vi "Pagina sinottico.vi"() -> (0 "pagina out":i16=255)   [LabVIEW 2022 SP3]
uses:
  Labview/Globali.vi
  <vilib>/Utility/inputDevices.llb/closeKeyboard.vi
  <vilib>/Utility/inputDevices.llb/keyboardAcquire.vi
panel:
  in  "solo a macchina ferma e ciclo concluso":bool
  out "CARRO IN POSIZIONE RP3000":bool
  out "CARRO IN POSIZIONE AAT":bool
  out "PRESSURIZZAZIONE":sgl(slide) caption="Pressurizz.\n\n[bar]" scale=0.0..1.0 scale format="%.1f"
  out "PRESSIONE ARIA 6 BAR":sgl(slide) caption="Pressione\n\n[bar]" scale=0.0..10.0
  out "PORTATA RICIRCOLO":sgl(slide) caption="Portata\nricircolo\n[l/min]" scale=0.0..25.0
  out "Cicli macchina":u16 caption="TIMEOUT\nMANUTENZIONE"
  in  "Vi/NaSH+F2":bool
  in  "Continua prova":bool
  in  "SOSPENDI PROVA":bool
  out "TEMPERATURA OLIO 10W30":sgl(slide) caption="Temperatura olio 10W30 [°C]" scale=0.0..100.0
  out "TEMPERATURA OLIO W90":sgl(slide) caption="Temperatura olio W90 [°C]" scale=0.0..100.0
  out "Rotaz.SX":bool
  out "Rotaz.DX":bool
  out "VELOCITA' MOTORE":u16(knob) caption="Velocità\n[rpm]" scale=0.0..3000.0
  out "Serial Number":string
  out "Prodotto":string
  in  "ANNULLA PROVA":bool
  out "S_AUTO":bool
  in  "0. 1":bool
  out "AVANZAMENTO COLLAUDO":i8(slide) scale=0.0..8.0
  out "t. 7":i32=17395251 format="%<%H:%M:%S>t"
  out "t. 6":i32=17395251 format="%<%H:%M:%S>t"
  out "t. 5":i32=17395251 format="%<%H:%M:%S>t"
  out "t. 4":i32=17395251 format="%<%H:%M:%S>t"
  out "t. 3":i32=17395251 format="%<%H:%M:%S>t"
  out "t. 2":i32=17395251 format="%<%H:%M:%S>t"
  out "t. 1":i32=17395251 format="%<%H:%M:%S>t"
  in  "t. 0":i32=17395251 format="%<%H:%M:%S>t"
  in  "Si/No 9":cluster{"Si":bool, "No":bool}
  in  "Si/No 8":cluster{"Si":bool, "No":bool}
  in  "Si/No 7":cluster{"Si":bool, "No":bool}
  in  "Si/No 6":cluster{"Si":bool, "No":bool}
  in  "Si/No 5":cluster{"Si":bool, "No":bool}
  in  "Si/No 4":cluster{"Si":bool, "No":bool}
  in  "Si/No 3":cluster{"Si":bool, "No":bool}
  in  "Si/No 2":cluster{"Si":bool, "No":bool}
  in  "Si/No 1":cluster{"Si":bool, "No":bool}
  out "t. tot.":i32 format="%<%H:%M:%S>t"
  out "t. Step":i32 format="%<%H:%M:%S>t"
  out "Indicazioni":string="Operatore:\t\t\t\t\t\t\t\t\t\t\t\t\t\t\t\t\t\t\t\t\t\t\t\t\t\t\t\t\t\t\t\tPart number:\t\t\t\t\t\t\t\t\t\t\t\t\t\t\t\t\t\t\t\t\t\t\t\t\t\t\t\t\t\t\t\tMatricola:\t\t\t\t\t\t\t\t\t\t\t\t\t\t\t\t0\t\t\t\t\t\t\t\t\t\t\t\t\t\t\t\tStatus \t\t\t\t\t\t\t\t\t\t\t\t\t\t\t\tC:\\Documents and Settings\\IVECO\\Reports\\\\"
  out "Prova":bool=TRUE
  in  "Login":bool
  in  "stop":bool
  in  "Comandi manuali":bool
  out "Picture":picture
  out "Versione SW":dbl=2.0 format="%.2f"
  out "Linea":string="BANCO PROVA TENUTA"
  out "Tipo pagina":string="PROVA"
  out "PRESSIONE RICIRCOLO":sgl(slide) caption="Pressione\nricircolo\n[bar]" scale=0.0..2.5 scale format="%.1f"
  out "TEMPERATURA CUSCIN.":sgl(slide) caption="Temperatura\ncuscinetto\n[°C]" scale=0.0..120.0
  out "TEMPERATURA OLIO COPPA":sgl(slide) caption="Temperatura\nolio coppa\n[°C]" scale=0.0..120.0
  out "COPPIA ASSE":sgl(knob) caption="Coppia\n[Nm]" scale=0.0..100.0
  out "Trazione inserita":bool
  out "PROT35":bool
  out "W90":bool
  out "10W30":bool
  in  "2. 5":bool
  in  "1. 3":bool
  in  "2. 0":bool
  in  "2. 3":bool
  in  "1. 4":bool
  in  "1. 5":bool
  in  "1. 6":bool
  in  "1. 7":bool
  in  "2. 1":bool
  in  "2. 2":bool
  in  "2. 4":bool
  out "TEMPERATURA AMBIENTE":sgl(slide) caption="Temperatura\nambiente\n[°C]" scale=0.0..50.0
  in  "1. 1":bool
  in  "1. 2":bool
  in  "0. 7":bool
  in  "1. 0":bool
  in  "0. 5":bool
  in  "0. 6":bool
  in  "0. 2":bool
  in  "0. 3":bool
  in  "0. 4":bool
  out "Testo allarmi":string caption="ALLARMI"
  out "Testo fase collaudo":string caption="FASE COLLAUDO"
  out "Testo segnalazioni":string caption="SEGNALAZIONI"
  out "Testo messaggi":string caption="MESSAGGI"
  out "forza chiusura":bool
  out "PLC->PC":string[](array[string])
  out "COD.PRODOTTO":string
  out "CODICE":string
  out "MATRICOLA OPERATORE":string
  in  "Pagina misure":bool
  in  "stop 2":bool
  in  "Pagina diagnostica":bool
  in  "Pagina scarti":bool
  out "Nome File Dati":string="C:\\Documents and Settings\\IVECO\\Reports\\\\"
  in  "Pagina parametri":bool
  out "operazioni":string[][](table)
  # "MODO FUNZIONAMENTO"
  # "INSERIMENTO TRAZIONE"
  # "SELETTORE SCARICO"
  # "OPERAZIONE"
  # "RICIRCOLO OLIO"
  # "CARICO/SCARICO PRESSURIZZAZIONE"
  # "CARICO/SCARICO ARIA"
  # "MOTORE"
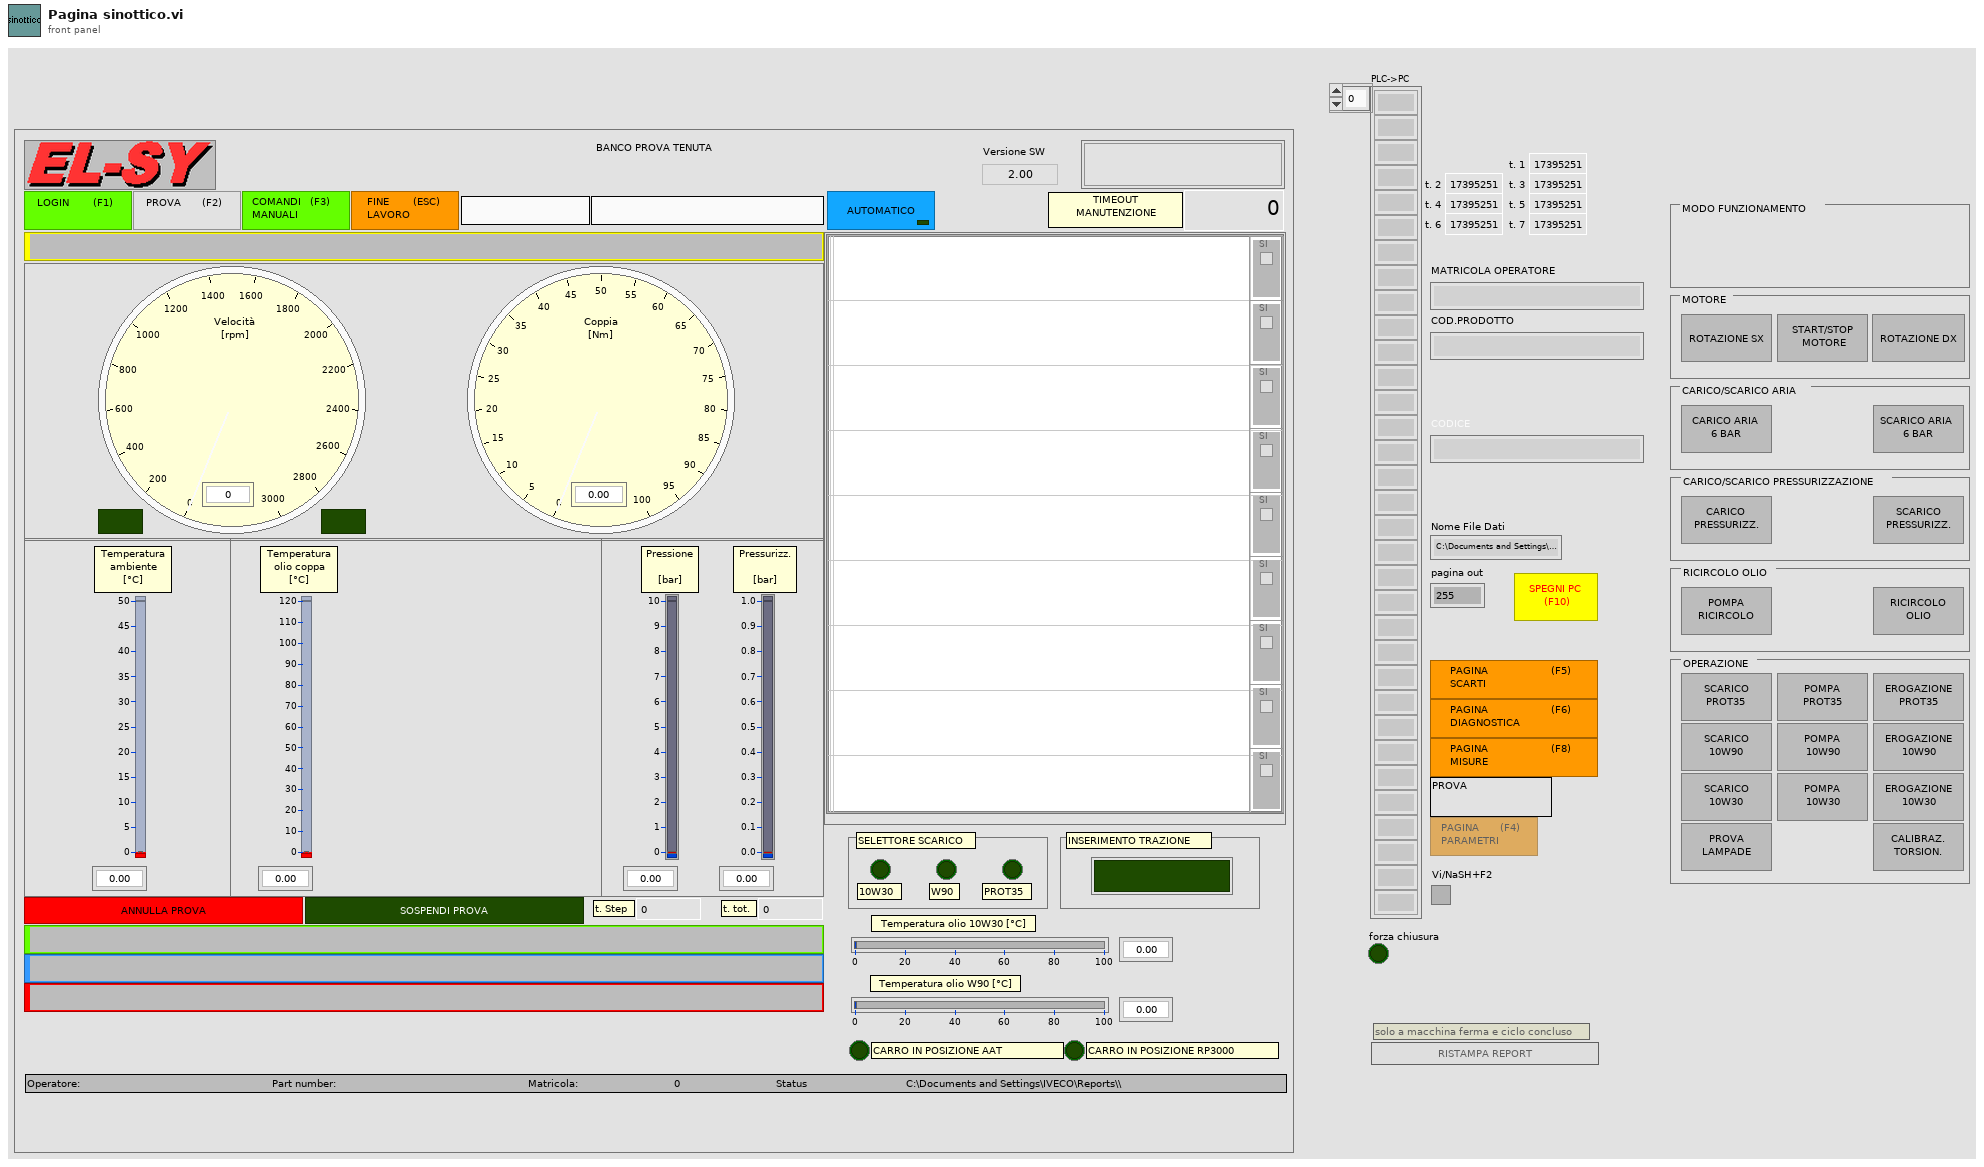
[diagram p1: front panel]
types:
  T1 = enum16{"0", "1", "2", "3", "4", "5", "6", "7", "8", "9", "A", "B", "C", "D", "E", "F", "G", "H", "I", "J", "K", "L", "M", "N", "O", "P", "Q", "R", "S", "T", "U", "V", "W", "X", "Y", "Z", "F1", "F2", "F3", "F4", "F5", "F6", "F7", "F8", "F9", "F10", "F11", "F12", "F13", "F14", "F15", "ADD", "BACK", "BACKSLASH", "CAPITAL", "COMMA", "DECIMAL", "DELETE", "DIVIDE", "DOWN", "END", "EQUALS", "ESCAPE", "GRAVE (`)", "HOME", "INSERT", "LBRACKET", "LCONTROL", "LEFT", "L ALT", "LSHIFT", "LWIN", "MINUS", "MULTIPLY", "NEXT", "NUMLOCK", "NUMPAD_0", "NUMPAD_1", "NUMPAD_2", "NUMPAD_3", "NUMPAD_4", "NUMPAD_5", "NUMPAD_6", "NUMPAD_7", "NUMPAD_8", "NUMPAD_9", "PAUSE", "PERIOD", "PRIOR (PG UP)", "RBRACKET", "RCONTROL", "RETURN", "RIGHT", "R ALT", "RSHIFT", "RWIN", "SCROLL", "SEMICOLON", "SLASH", "SPACE", "SUBTRACT", "TAB", "UP", "ENTER (num pad)", "' (quote)"}[]
  T2 = cluster{"Disable?":i16, "Si":bool, "No":bool, "Dis. No?":i16}
  T3 = enum16{"0", "1", "2", "3", "4", "5", "6", "7", "8", "9", "A", "B", "C", "D", "E", "F", "G", "H", "I", "J", "K", "L", "M", "N", "O", "P", "Q", "R", "S", "T", "U", "V", "W", "X", "Y", "Z", "F1", "F2", "F3", "F4", "F5", "F6", "F7", "F8", "F9", "F10", "F11", "F12", "F13", "F14", "F15", "ADD", "BACK", "BACKSLASH", "CAPITAL", "COMMA", "DECIMAL", "DELETE", "DIVIDE", "DOWN", "END", "EQUALS", "ESCAPE", "GRAVE (`)", "HOME", "INSERT", "LBRACKET", "LCONTROL", "LEFT", "L ALT", "LSHIFT", "LWIN", "MINUS", "MULTIPLY", "NEXT", "NUMLOCK", "NUMPAD_0", "NUMPAD_1", "NUMPAD_2", "NUMPAD_3", "NUMPAD_4", "NUMPAD_5", "NUMPAD_6", "NUMPAD_7", "NUMPAD_8", "NUMPAD_9", "PAUSE", "PERIOD", "PRIOR (PG UP)", "RBRACKET", "RCONTROL", "RETURN", "RIGHT", "R ALT", "RSHIFT", "RWIN", "SCROLL", "SEMICOLON", "SLASH", "SPACE", "SUBTRACT", "TAB", "UP", "ENTER (num pad)", "' (quote)"}
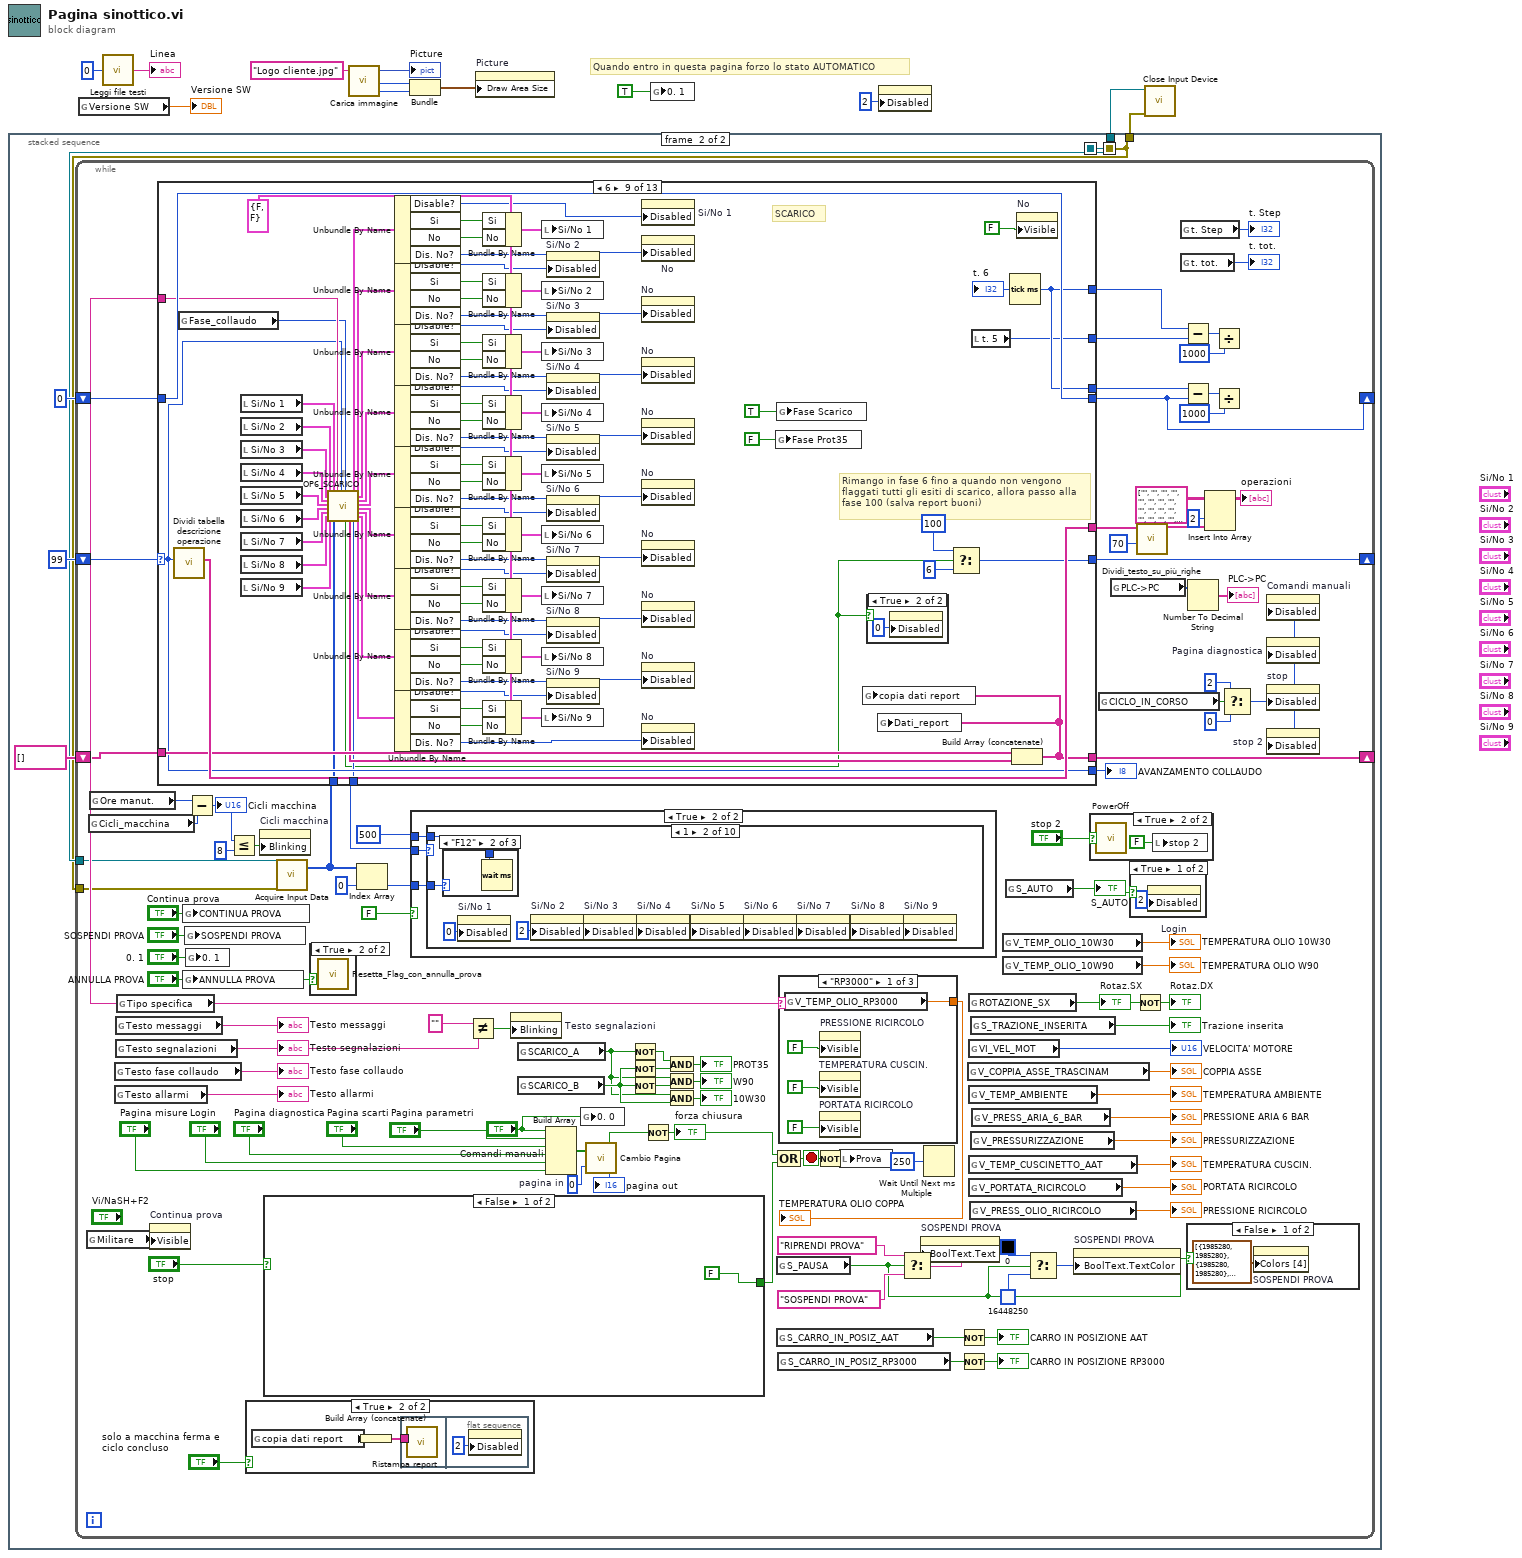
[diagram p0: block diagram]
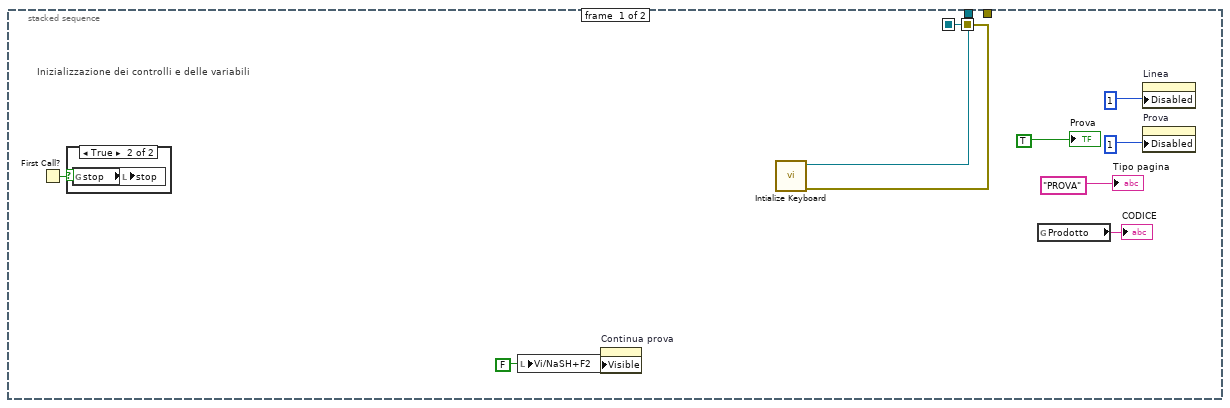
[diagram p2: hidden frame]
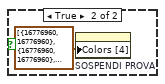
[diagram p5: hidden frame]
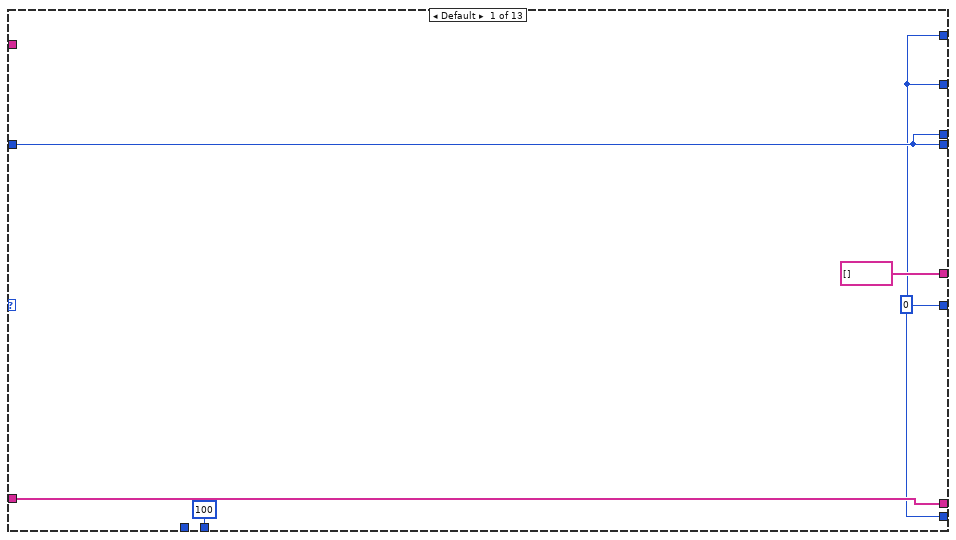
[diagram p6: hidden frame]
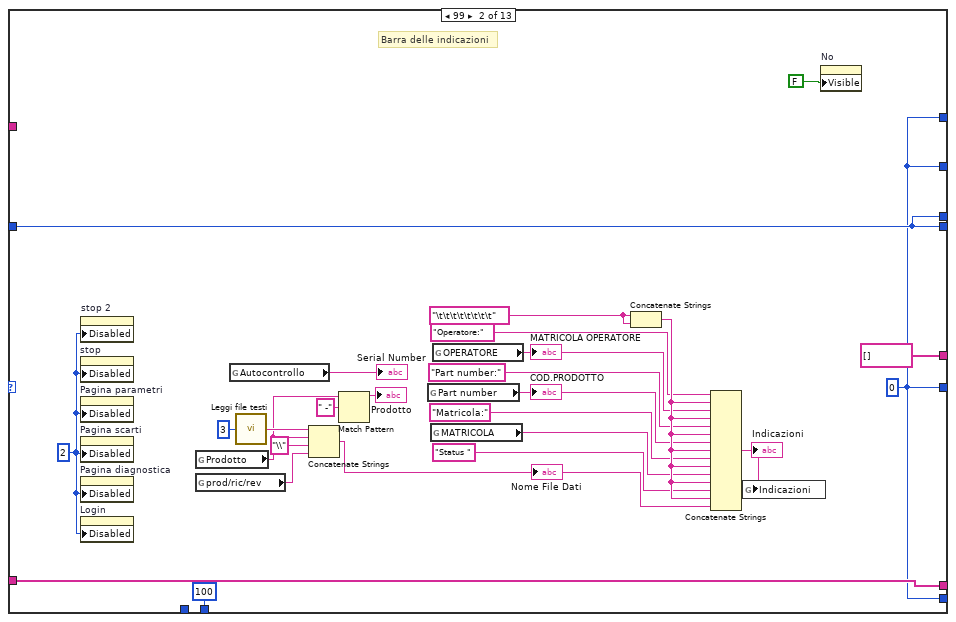
[diagram p7: hidden frame]
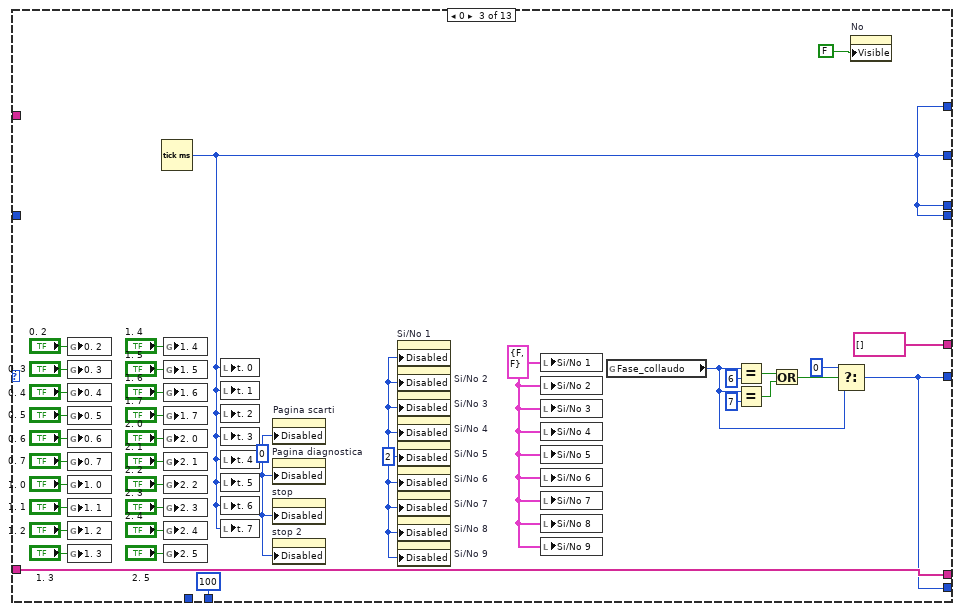
[diagram p8: hidden frame]
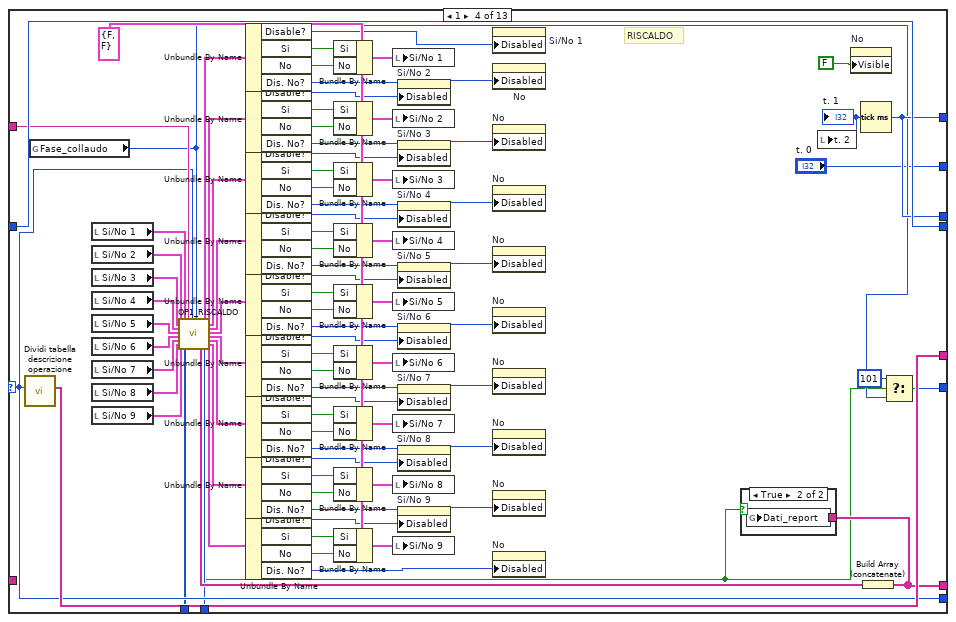
[diagram p9: hidden frame]
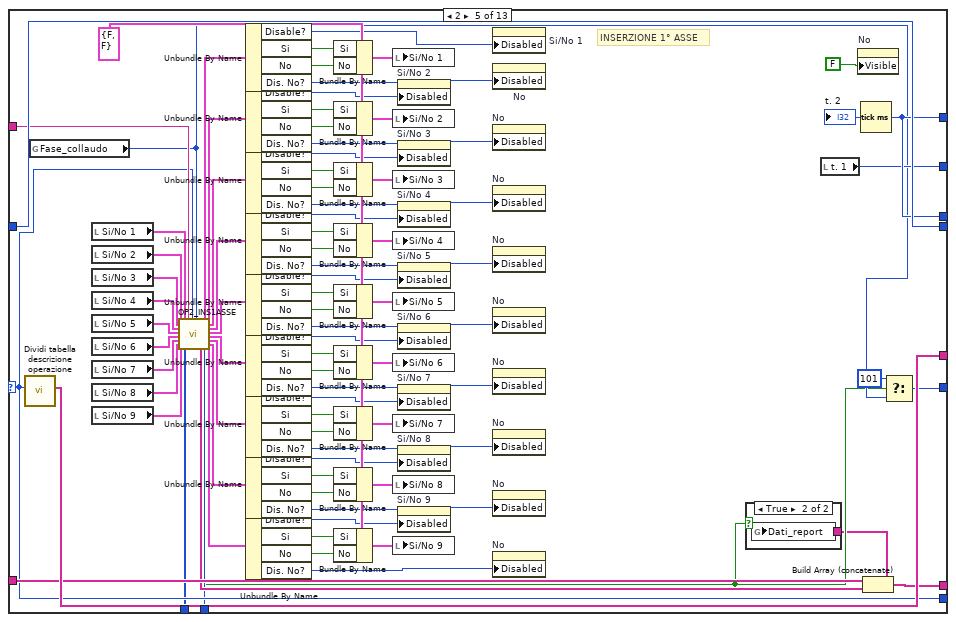
[diagram p11: hidden frame]
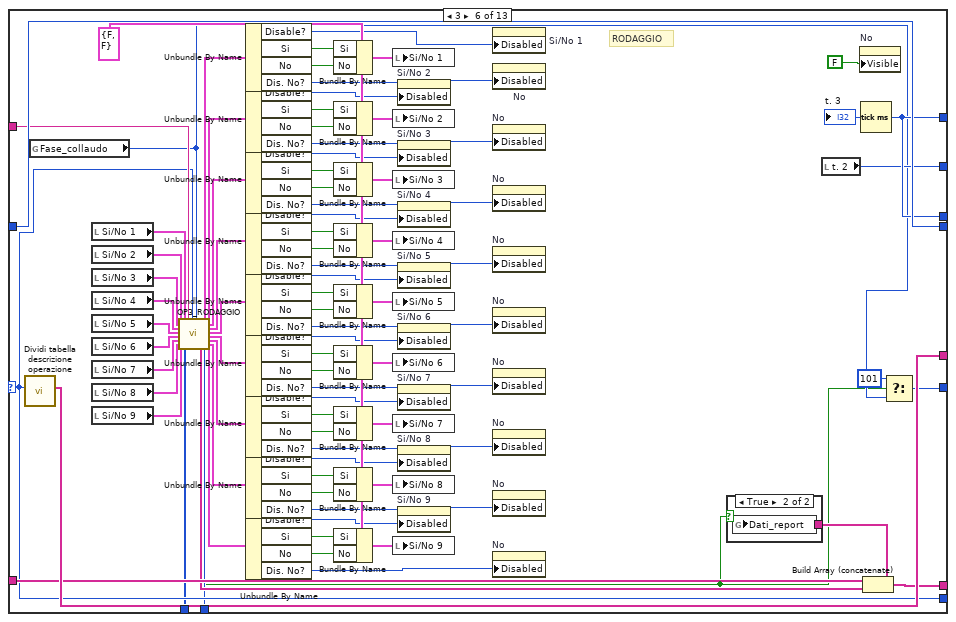
[diagram p13: hidden frame]
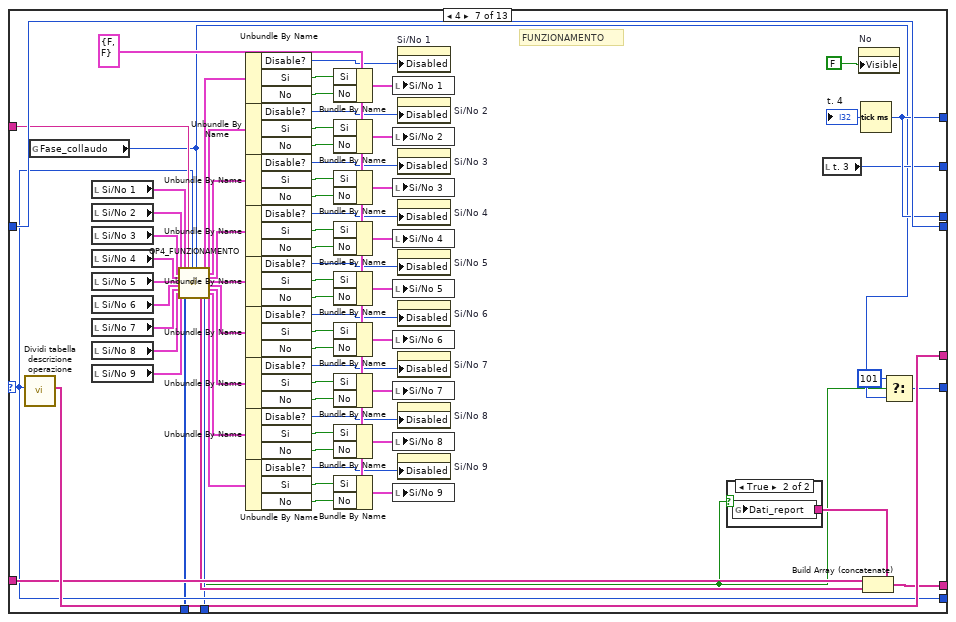
[diagram p15: hidden frame]
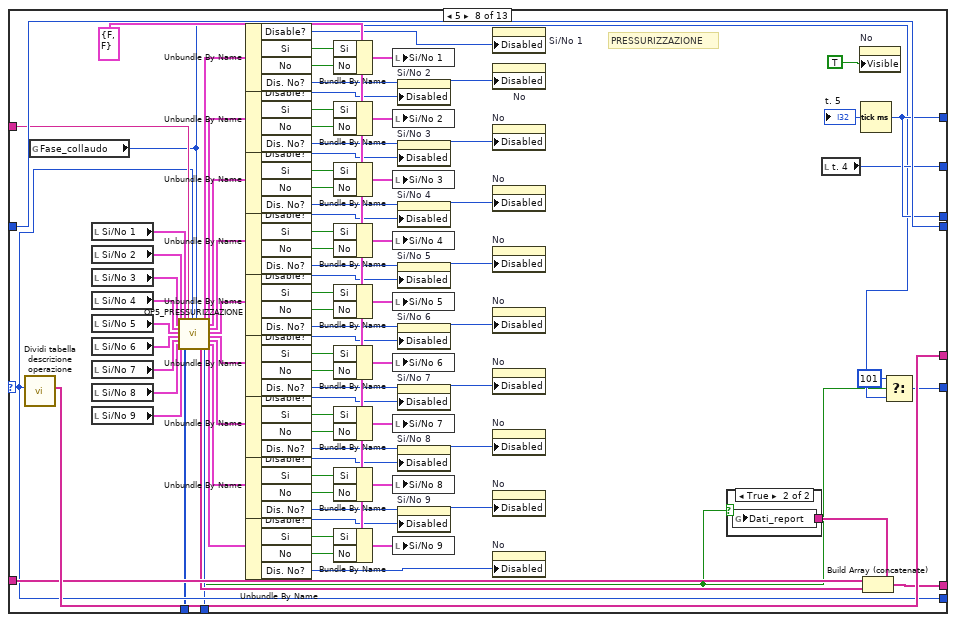
[diagram p17: hidden frame]
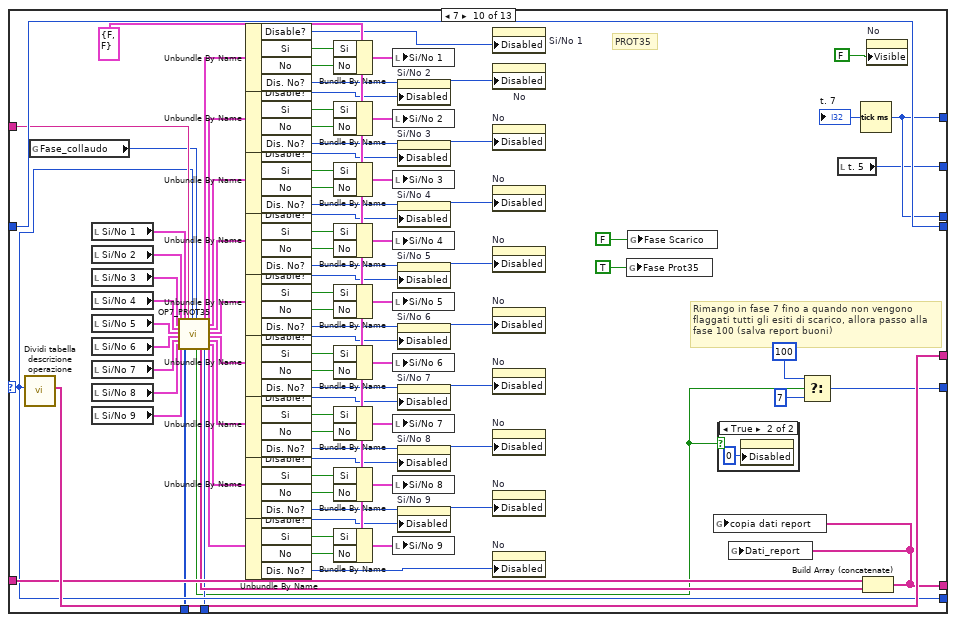
[diagram p20: hidden frame]
diagram:
  # "Quando entro in questa pagina forzo lo stato AUTOMATICO"
  n1 = stacked-sequence {
    seq-local: [w16 _] -> [_ w24]
    seq-local: [w15 _] -> [_ w23]
    tunnel: [_ w23] -> w12
    tunnel: [_ w24] -> w11
    frame #0 {
      w13 = FALSE ("Vi/NaSH+F2")
      # "Inizializzazione dei controlli e delle variabili"
      n2 = First Call?() -> (First Call?: T/F=w21:bool)
      n3 = case shown="True" w21 {
        frame False {
        }
        frame True {
          n4 = global read "Globali.vi" "stop"() -> (w22:bool)
          n5 = local write "stop"(w22) -> ()
        }
      }
      n6 = local write "Vi/NaSH+F2"(w13) -> ()
      n7 = property on="Continua prova" class="Bool (strict)"("Visible"=w13) -> ()  [unwired: 2 in, 2 out]
      n8 = call <vilib>:"Intialize Keyboard.vi"() -> ("error out"=w15:errorcluster, "device ID"=w16:refnum<k1>)  [unwired: 10 in]
      n9 = global read "Globali.vi" "Prodotto"() -> (→"CODICE":string)
      n10 = property on="Linea" class="Str"("Disabled"=u8 1) -> ()  [unwired: 2 in, 2 out]
      n11 = property on="Prova" class="Bool"("Disabled"=u8 1) -> ()  [unwired: 2 in, 2 out]
      "Prova" <- TRUE ("Pagina sinottico")
      "Tipo pagina" <- "PROVA" ("Tipo pagina")
    }
    frame #1 {
      n12 = while {
        shift-right: [w103] -> _
        shift-left: 99 ("Fase_collaudo") -> [w132]
        shift-right: [w101] -> _
        shift-left: u32 0 ("millisecond timer value") -> [w102]
        shift-right: [w96] -> _
        shift-left: string[] [] -> [w95]
        tunnel: w24 -> [w90]
        tunnel: w23 -> [w89]
        stop <- w105 stop-if-true
        w129 = u8 0  # pagina in
        n13 = global read "Globali.vi" "Militare"() -> (w45:bool)
        n14 = global read "Globali.vi" "Cicli_macchina"() -> (w39:u16)
        n15 = global read "Globali.vi" "Ore manut."() -> (w40:i16)
        n16 = global read "Globali.vi" "Testo fase collaudo"() -> (→"Testo fase collaudo":string)
        n17 = global read "Globali.vi" "Testo allarmi"() -> (→"Testo allarmi":string)
        n18 = global read "Globali.vi" "Testo messaggi"() -> (→"Testo messaggi":string)
        n19 = global read "Globali.vi" "Testo segnalazioni"() -> (w30:string)
        "Testo segnalazioni" <- w30
        n20 = global read "Globali.vi" "Tipo specifica"() -> (w97:string)
        n21 = property on="Continua prova" class="Bool (strict)"("Visible"=w45) -> ()  [unwired: 2 in, 2 out]
        n22 = global write "Globali.vi" "CONTINUA PROVA"("Continua prova") -> ()
        n23 = global write "Globali.vi" "ANNULLA PROVA"("ANNULLA PROVA") -> ()
        n24 = global write "Globali.vi" "SOSPENDI PROVA"("SOSPENDI PROVA") -> ()
        n25 = global write "Globali.vi" "0. 1"("0. 1") -> ()
        n26 = Subtract(x=w40, y=w39) -> (x-y=w38:u16)
        "Cicli macchina" <- w38
        n27 = Less Or Equal?(x=w38, y=u16 8) -> (x <= y?=w36:bool)
        n28 = case shown="True" "solo a macchina ferma e ciclo concluso" {
          frame False {
          }
          frame True {
            n29 = global read "Globali.vi" "copia dati report"() -> (w134:string[])
            n30 = Build Array (concatenate)(w134) -> (w133:string[])
            n31 = flat-sequence {
              tunnel: w133 -> [w135]
              frame #0 {
                n32 = call "Ristampa report.vi"("Dato"=w135) -> ()  [unwired: 7 in, 2 out]
              }
              frame #1 {
                n33 = property on="solo a macchina ferma e ciclo concluso" class="Bool"("Disabled"=u8 2) -> ()  [unwired: 2 in, 2 out]
              }
            }
          }
        }
        n34 = property on="Cicli macchina" class="DigNum (strict)"("Blinking"=w36) -> ()  [unwired: 2 in, 2 out]
        n35 = case shown="False" "stop" {
          tunnel: [FALSE ("x = y?") w893] -> w122
          frame False {
          }
          frame True {
            # "Quando esco dal programma forzo lo stato MANUALE"
            n36 = Two Button Dialog(message="USCIRE DALL'APPLICAZIONE?" ("T button name (\"OK\")"), 1:"NO" ("F button name (\"Cancel\")"), 2:"SI" ("T button name (\"OK\")")) -> (T button?=w896:bool)
            n37 = Select(t=TRUE, s=w896, f=FALSE) -> (s? t:f=w894:bool)
            n38 = case shown="True" w894 {
              tunnel: [FALSE ("S_MAN") w902] -> w893
              frame False {
              }
              frame True {
                n39 = while {
                  tunnel: [w903] -> w902
                  stop <- w903 stop-if-true
                  n40 = global read "Globali.vi" "S_MAN"() -> (w903:bool)
                  n41 = Wait Until Next ms Multiple(millisecond multiple=u32 50) -> ()  [unwired: 1 out]
                }
              }
            }
            n42 = global write "Globali.vi" "0. 0"(w894) -> ()
            n43 = local write "stop"(w894) -> ()
            n44 = Quit LabVIEW(quit? (T)=w893) -> ()
            n45 = global write "Globali.vi" "stop"(w893) -> ()
          }
        }
        n46 = call-poly <vilib>:"Acquire Input Data.vi"("device ID"=w90, "error in (no error)"=w89) -> ("keys pressed"=w87:T1)  [unwired: 15 in, 2 out]
        n47 = case shown="6" w132 {
          selector: w132 -> [_ _ _ w215 w294 w375 w456 w528 w610 w695 _ _ _]
          tunnel: [w140 w153 w172 w211 w289 w370 w451 w523 w604 w687 w774 w797 w815] -> w103
          tunnel: [w140 w153 w179 w216 w296 w377 w458 w530 w612 w697 w783 w806 w815] -> w73
          tunnel: [w140 w153 w179 "t. 0" w295 w376 w457 w529 w611 w696 w777 w800 w815] -> w61
          tunnel: [string[] [] string[] [] string[] [] w246 w327 w408 w480 w561 w645 w729 string[] [] string[] [] string[] [] ("operazioni")] -> w64
          tunnel: [w142 w167 w179 w247 w328 w409 w481 w562 w646 w730 w784 w807 w816] -> w101
          tunnel: w102 -> [w142 w167 _ w247 w328 w409 w481 w562 w646 w730 w784 w807 w816]
          tunnel: [w142 w167 w179 w216 w296 w377 w458 w530 w612 w697 w783 w806 w816] -> w65
          tunnel: w97 -> [_ _ _ w236 w317 w398 w470 w551 w635 w719 w769 w792 _]
          tunnel: [w141 w166 w184 w207 w286 w368 w449 w521 w605 w691 w772 w795 w818] -> w96
          tunnel: w95 -> [w141 w166 w184 _ w298 w379 w460 w532 w616 w699 _ _ w818]
          tunnel: [w140 w153 w172 w215 w294 w375 w456 w528 w610 w695 8 ("Fase_collaudo") 8 ("Fase_collaudo") w815] -> w60
          tunnel: [100 ("i out") 100 ("i out") 100 ("i out") w214 w293 w373 w455 w527 w609 w694 100 ("i out") 100 ("i out") 100 ("i out")] -> w88
          tunnel: w87 -> [_ _ _ w213 w292 w374 w454 w526 w608 w693 _ _ _]
          frame Default {
            w140 = 0
          }
          frame 99 {
            w163 = "\t\t\t\t\t\t\t\t" ("String")
            w169 = u8 2 ("Disabled")
            w153 = 0
            # "Barra delle indicazioni"
            n48 = property on="stop 2" class="Bool (strict)"("Disabled"=w169) -> ()  [unwired: 2 in, 2 out]
            n49 = property on="stop" class="Bool (strict)"("Disabled"=w169) -> ()  [unwired: 2 in, 2 out]
            n50 = property on="Pagina parametri" class="Bool"("Disabled"=w169) -> ()  [unwired: 2 in, 2 out]
            n51 = property on="Pagina scarti" class="Bool"("Disabled"=w169) -> ()  [unwired: 2 in, 2 out]
            n52 = property on="Pagina diagnostica" class="Bool"("Disabled"=w169) -> ()  [unwired: 2 in, 2 out]
            n53 = property on="Login" class="Bool"("Disabled"=w169) -> ()  [unwired: 2 in, 2 out]
            n54 = global read "Globali.vi" "Prodotto"() -> (w150:string)
            n55 = global read "Globali.vi" "prod/ric/rev"() -> (w146:string)
            n56 = global read "Globali.vi" "Autocontrollo"() -> (→"Serial Number":string)
            n57 = call "Leggi file testi.vi"("Numero riga"=3) -> ("Testo"=w165:string)  [unwired: 3 in, 1 out]
            n58 = Concatenate Strings(w165, w150, "\\" ("string"), w146) -> (w144:string)
            "Nome File Dati" <- w144
            n59 = Match Pattern(string=w150, regular expression=" -") -> (before substring=→"Prodotto":string)  [unwired: 1 in, 3 out]
            n60 = global read "Globali.vi" "Part number"() -> (w161:string)
            "COD.PRODOTTO" <- w161
            n61 = global read "Globali.vi" "MATRICOLA"() -> (w160:string)
            n62 = global read "Globali.vi" "OPERATORE"() -> (w159:string)
            "MATRICOLA OPERATORE" <- w159
            n63 = Concatenate Strings(w163, w163) -> (w162:string)
            n64 = Concatenate Strings("Operatore:" ("string"), w162, w159, w162, "Part number:" ("string"), w162, w161, w162, "Matricola:" ("string"), w162, w160, w162, "Status " ("string"), w162, w144) -> (w154:string)
            "Indicazioni" <- w154
            n65 = global write "Globali.vi" "Indicazioni"(w154) -> ()
            n66 = property on="No" class="Bool (strict)"("Visible"=FALSE) -> ()  [unwired: 2 in, 2 out]
          }
          frame 0 {
            w180 = cluster{"Si":bool, "No":bool} {"Si"=FALSE, "No"=FALSE} ("Si/No 1")
            w182 = u8 0 ("Disabled")
            w183 = 2
            n67 = global write "Globali.vi" "0. 2"("0. 2") -> ()
            n68 = global write "Globali.vi" "0. 3"("0. 3") -> ()
            n69 = global write "Globali.vi" "0. 4"("0. 4") -> ()
            n70 = global write "Globali.vi" "0. 5"("0. 5") -> ()
            n71 = global write "Globali.vi" "0. 6"("0. 6") -> ()
            n72 = global write "Globali.vi" "0. 7"("0. 7") -> ()
            n73 = global write "Globali.vi" "1. 0"("1. 0") -> ()
            n74 = global write "Globali.vi" "1. 1"("1. 1") -> ()
            n75 = global write "Globali.vi" "1. 2"("1. 2") -> ()
            n76 = global write "Globali.vi" "1. 3"("1. 3") -> ()
            n77 = Tick Count (ms)() -> (millisecond timer value=w179:u32)
            n78 = global write "Globali.vi" "1. 4"("1. 4") -> ()
            n79 = global write "Globali.vi" "1. 5"("1. 5") -> ()
            n80 = global write "Globali.vi" "1. 6"("1. 6") -> ()
            n81 = global write "Globali.vi" "1. 7"("1. 7") -> ()
            n82 = global write "Globali.vi" "2. 0"("2. 0") -> ()
            n83 = global write "Globali.vi" "2. 1"("2. 1") -> ()
            n84 = global write "Globali.vi" "2. 2"("2. 2") -> ()
            n85 = global write "Globali.vi" "2. 3"("2. 3") -> ()
            n86 = global write "Globali.vi" "2. 4"("2. 4") -> ()
            n87 = global write "Globali.vi" "2. 5"("2. 5") -> ()
            n88 = local write "t. 0"(w179) -> ()
            n89 = local write "t. 1"(w179) -> ()
            n90 = local write "t. 2"(w179) -> ()
            n91 = local write "t. 3"(w179) -> ()
            n92 = local write "t. 4"(w179) -> ()
            n93 = local write "t. 5"(w179) -> ()
            n94 = local write "t. 6"(w179) -> ()
            n95 = local write "t. 7"(w179) -> ()
            n96 = property on="Pagina scarti" class="Bool"("Disabled"=w182) -> ()  [unwired: 2 in, 2 out]
            n97 = property on="Pagina diagnostica" class="Bool"("Disabled"=w182) -> ()  [unwired: 2 in, 2 out]
            n98 = property on="stop" class="Bool (strict)"("Disabled"=w182) -> ()  [unwired: 2 in, 2 out]
            n99 = property on="stop 2" class="Bool (strict)"("Disabled"=w182) -> ()  [unwired: 2 in, 2 out]
            n100 = property on="Si/No 1" class="Clust (strict)"("Disabled"=w183) -> ()  [unwired: 2 in, 2 out]
            n101 = property on="Si/No 2" class="Clust (strict)"("Disabled"=w183) -> ()  [unwired: 2 in, 2 out]
            n102 = property on="Si/No 3" class="Clust (strict)"("Disabled"=w183) -> ()  [unwired: 2 in, 2 out]
            n103 = property on="Si/No 4" class="Clust (strict)"("Disabled"=w183) -> ()  [unwired: 2 in, 2 out]
            n104 = property on="Si/No 5" class="Clust (strict)"("Disabled"=w183) -> ()  [unwired: 2 in, 2 out]
            n105 = property on="Si/No 6" class="Clust (strict)"("Disabled"=w183) -> ()  [unwired: 2 in, 2 out]
            n106 = property on="Si/No 7" class="Clust (strict)"("Disabled"=w183) -> ()  [unwired: 2 in, 2 out]
            n107 = property on="Si/No 8" class="Clust (strict)"("Disabled"=w183) -> ()  [unwired: 2 in, 2 out]
            n108 = property on="Si/No 9" class="Clust (strict)"("Disabled"=w183) -> ()  [unwired: 2 in, 2 out]
            n109 = local write "Si/No 1"(w180) -> ()
            n110 = local write "Si/No 2"(w180) -> ()
            n111 = local write "Si/No 3"(w180) -> ()
            n112 = local write "Si/No 4"(w180) -> ()
            n113 = local write "Si/No 5"(w180) -> ()
            n114 = local write "Si/No 6"(w180) -> ()
            n115 = local write "Si/No 7"(w180) -> ()
            n116 = local write "Si/No 8"(w180) -> ()
            n117 = local write "Si/No 9"(w180) -> ()
            n118 = global read "Globali.vi" "Fase_collaudo"() -> (w170:u16)
            n119 = Equal?(x=w170, y=u16 6) -> (x = y?=w175:bool)
            n120 = Equal?(x=w170, y=u16 7) -> (x = y?=w174:bool)
            n121 = Or(x=w175, y=w174) -> (x .or. y?=w173:bool)
            n122 = Select(t=u16 0 ("y"), s=w173, f=w170) -> (s? t:f=w172:u16)
            n123 = property on="No" class="Bool (strict)"("Visible"=FALSE) -> ()  [unwired: 2 in, 2 out]
          }
          frame 1 {
            w278 = cluster{"Si":bool, "No":bool} {"Si"=FALSE, "No"=FALSE} ("Si/No 1")
            # "RISCALDO"
            n124 = call "Dividi tabella descrizione operazione.vi"("Numero operazione"=w215) -> ("operazioni"=w246:string[])  [unwired: 10 in]
            n125 = global read "Globali.vi" "Fase_collaudo"() -> (w212:u16)
            n126 = local read "Si/No 1"() -> (w245:cluster{"Si":bool, "No":bool})
            n127 = local read "Si/No 2"() -> (w244:cluster{"Si":bool, "No":bool})
            n128 = local read "Si/No 3"() -> (w243:cluster{"Si":bool, "No":bool})
            n129 = local read "Si/No 4"() -> (w242:cluster{"Si":bool, "No":bool})
            n130 = local read "Si/No 5"() -> (w241:cluster{"Si":bool, "No":bool})
            n131 = local read "Si/No 6"() -> (w237:cluster{"Si":bool, "No":bool})
            n132 = local read "Si/No 7"() -> (w238:cluster{"Si":bool, "No":bool})
            n133 = local read "Si/No 8"() -> (w239:cluster{"Si":bool, "No":bool})
            n134 = local read "Si/No 9"() -> (w240:cluster{"Si":bool, "No":bool})
            n135 = call "OP1_RISCALDO.vi"("Esito 2 in"=w244, "Esito 3 in"=w243, "Esito 4 in"=w242, "Esito 5 in"=w241, "Esito 6 in"=w237, "Esito 7 in"=w238, "Esito 8 in"=w239, "Esito 9 in"=w240, "Esito 1 in"=w245, "Tasto premuto"=w213, "Tipo specifica"=w236, "Stato in"=w215, "Stato out"=w212) -> ("Dato"=w217:string[], "ANNULLA PROVA"=w206:bool, "Esito 1 out"=w235:T2, "i out"=w214:i32, "Esito 2 out"=w234:T2, "Esito 3 out"=w233:T2, "Esito 4 out"=w232:T2, "Esito 5 out"=w231:T2, "Esito 6 out"=w227:T2, "Esito 7 out"=w228:T2, "Esito 8 out"=w229:T2, "Esito 9 out"=w230:T2)  [unwired: 3 in]
            n136 = Unbundle By Name(w235) -> ("Disable?"=w248:i16, "Si"=w249:bool, "No"=w250:bool, "Dis. No?"=w226:i16)
            n137 = Unbundle By Name(w234) -> ("Disable?"=w254:i16, "Si"=w253:bool, "No"=w252:bool, "Dis. No?"=w218:i16)
            n138 = Unbundle By Name(w233) -> ("Disable?"=w270:i16, "Si"=w259:bool, "No"=w258:bool, "Dis. No?"=w219:i16)
            n139 = Unbundle By Name(w232) -> ("Disable?"=w271:i16, "Si"=w256:bool, "No"=w257:bool, "Dis. No?"=w220:i16)
            n140 = Unbundle By Name(w231) -> ("Disable?"=w272:i16, "Si"=w267:bool, "No"=w266:bool, "Dis. No?"=w221:i16)
            n141 = Unbundle By Name(w227) -> ("Disable?"=w273:i16, "Si"=w264:bool, "No"=w265:bool, "Dis. No?"=w222:i16)
            n142 = Unbundle By Name(w228) -> ("Disable?"=w274:i16, "Si"=w260:bool, "No"=w261:bool, "Dis. No?"=w223:i16)
            n143 = Unbundle By Name(w229) -> ("Disable?"=w275:i16, "Si"=w263:bool, "No"=w262:bool, "Dis. No?"=w224:i16)
            n144 = Unbundle By Name(w230) -> ("Disable?"=w276:i16, "Si"=w268:bool, "No"=w269:bool, "Dis. No?"=w225:i16)
            n145 = Bundle By Name(cluster=w278, "Si"=w249, "No"=w250) -> (w251:cluster{"Si":bool, "No":bool})
            n146 = Bundle By Name(cluster=w278, "Si"=w253, "No"=w252) -> (w255:cluster{"Si":bool, "No":bool})
            n147 = Bundle By Name(cluster=w278, "Si"=w259, "No"=w258) -> (w284:cluster{"Si":bool, "No":bool})
            n148 = Bundle By Name(cluster=w278, "Si"=w256, "No"=w257) -> (w283:cluster{"Si":bool, "No":bool})
            n149 = Bundle By Name(cluster=w278, "Si"=w267, "No"=w266) -> (w282:cluster{"Si":bool, "No":bool})
            n150 = Bundle By Name(cluster=w278, "Si"=w264, "No"=w265) -> (w281:cluster{"Si":bool, "No":bool})
            n151 = Bundle By Name(cluster=w278, "Si"=w260, "No"=w261) -> (w280:cluster{"Si":bool, "No":bool})
            n152 = Bundle By Name(cluster=w278, "Si"=w263, "No"=w262) -> (w279:cluster{"Si":bool, "No":bool})
            n153 = Bundle By Name(cluster=w278, "Si"=w268, "No"=w269) -> (w277:cluster{"Si":bool, "No":bool})
            n154 = local write "Si/No 1"(w251) -> ()
            n155 = local write "Si/No 2"(w255) -> ()
            n156 = local write "Si/No 3"(w284) -> ()
            n157 = local write "Si/No 4"(w283) -> ()
            n158 = local write "Si/No 5"(w282) -> ()
            n159 = local write "Si/No 6"(w281) -> ()
            n160 = local write "Si/No 7"(w280) -> ()
            n161 = local write "Si/No 8"(w279) -> ()
            n162 = local write "Si/No 9"(w277) -> ()
            n163 = property on="Si/No 2" class="Clust (strict)"("Disabled"=w254) -> ()  [unwired: 2 in, 2 out]
            n164 = property on="Si/No 3" class="Clust (strict)"("Disabled"=w270) -> ()  [unwired: 2 in, 2 out]
            n165 = property on="Si/No 4" class="Clust (strict)"("Disabled"=w271) -> ()  [unwired: 2 in, 2 out]
            n166 = property on="Si/No 5" class="Clust (strict)"("Disabled"=w272) -> ()  [unwired: 2 in, 2 out]
            n167 = property on="Si/No 6" class="Clust (strict)"("Disabled"=w273) -> ()  [unwired: 2 in, 2 out]
            n168 = property on="Si/No 7" class="Clust (strict)"("Disabled"=w274) -> ()  [unwired: 2 in, 2 out]
            n169 = property on="Si/No 8" class="Clust (strict)"("Disabled"=w275) -> ()  [unwired: 2 in, 2 out]
            n170 = property on="Si/No 9" class="Clust (strict)"("Disabled"=w276) -> ()  [unwired: 2 in, 2 out]
            n171 = property on="Si/No 1" class="Clust (strict)"("Disabled"=w248) -> ()  [unwired: 2 in, 2 out]
            n172 = property on="No" class="Bool (strict)"("Disabled"=w226) -> ()  [unwired: 2 in, 2 out]
            n173 = property on="No" class="Bool (strict)"("Disabled"=w218) -> ()  [unwired: 2 in, 2 out]
            n174 = property on="No" class="Bool (strict)"("Disabled"=w219) -> ()  [unwired: 2 in, 2 out]
            n175 = property on="No" class="Bool (strict)"("Disabled"=w220) -> ()  [unwired: 2 in, 2 out]
            n176 = property on="No" class="Bool (strict)"("Disabled"=w221) -> ()  [unwired: 2 in, 2 out]
            n177 = property on="No" class="Bool (strict)"("Disabled"=w222) -> ()  [unwired: 2 in, 2 out]
            n178 = property on="No" class="Bool (strict)"("Disabled"=w223) -> ()  [unwired: 2 in, 2 out]
            n179 = property on="No" class="Bool (strict)"("Disabled"=w224) -> ()  [unwired: 2 in, 2 out]
            n180 = property on="No" class="Bool (strict)"("Disabled"=w225) -> ()  [unwired: 2 in, 2 out]
            n181 = property on="No" class="Bool (strict)"("Visible"=FALSE) -> ()  [unwired: 2 in, 2 out]
            n182 = Tick Count (ms)() -> (millisecond timer value=w216:u32)
            "t. 1" <- w216
            n183 = local write "t. 2"(w216) -> ()
            n184 = Build Array (concatenate)(w217) -> (w207:string[])
            n185 = case shown="True" w206 {
              tunnel: w207 -> [_ w285]
              frame False {
              }
              frame True {
                n186 = global write "Globali.vi" "Dati_report"(w285) -> ()
              }
            }
            n187 = Select(t=u16 101, s=w206, f=w212) -> (s? t:f=w211:u16)
          }
          frame 2 {
            w359 = cluster{"Si":bool, "No":bool} {"Si"=FALSE, "No"=FALSE} ("Si/No 1")
            # "INSERZIONE 1° ASSE"
            n188 = call "Dividi tabella descrizione operazione.vi"("Numero operazione"=w294) -> ("operazioni"=w327:string[])  [unwired: 10 in]
            n189 = global read "Globali.vi" "Fase_collaudo"() -> (w290:u16)
            n190 = local read "Si/No 1"() -> (w326:cluster{"Si":bool, "No":bool})
            n191 = local read "Si/No 2"() -> (w325:cluster{"Si":bool, "No":bool})
            n192 = local read "Si/No 3"() -> (w324:cluster{"Si":bool, "No":bool})
            n193 = local read "Si/No 4"() -> (w323:cluster{"Si":bool, "No":bool})
            n194 = local read "Si/No 5"() -> (w322:cluster{"Si":bool, "No":bool})
            n195 = local read "Si/No 6"() -> (w318:cluster{"Si":bool, "No":bool})
            n196 = local read "Si/No 7"() -> (w319:cluster{"Si":bool, "No":bool})
            n197 = local read "Si/No 8"() -> (w320:cluster{"Si":bool, "No":bool})
            n198 = local read "Si/No 9"() -> (w321:cluster{"Si":bool, "No":bool})
            n199 = call "OP2_INS1ASSE.vi"("Esito 2 in"=w325, "Esito 3 in"=w324, "Esito 4 in"=w323, "Esito 5 in"=w322, "Esito 6 in"=w318, "Esito 7 in"=w319, "Esito 8 in"=w320, "Esito 9 in"=w321, "Esito 1 in"=w326, "Tasto premuto"=w292, "Tipo specifica"=w317, "Stato in"=w294, "Stato out"=w290) -> ("Dato"=w297:string[], "ANNULLA PROVA"=w287:bool, "Esito 1 out"=w316:T2, "i out"=w293:i32, "Esito 2 out"=w315:T2, "Esito 3 out"=w314:T2, "Esito 4 out"=w313:T2, "Esito 5 out"=w312:T2, "Esito 6 out"=w308:T2, "Esito 7 out"=w309:T2, "Esito 8 out"=w310:T2, "Esito 9 out"=w311:T2)  [unwired: 3 in]
            n200 = Unbundle By Name(w316) -> ("Disable?"=w329:i16, "Si"=w330:bool, "No"=w331:bool, "Dis. No?"=w307:i16)
            n201 = Unbundle By Name(w315) -> ("Disable?"=w335:i16, "Si"=w334:bool, "No"=w333:bool, "Dis. No?"=w299:i16)
            n202 = Unbundle By Name(w314) -> ("Disable?"=w351:i16, "Si"=w340:bool, "No"=w339:bool, "Dis. No?"=w300:i16)
            n203 = Unbundle By Name(w313) -> ("Disable?"=w352:i16, "Si"=w337:bool, "No"=w338:bool, "Dis. No?"=w301:i16)
            n204 = Unbundle By Name(w312) -> ("Disable?"=w353:i16, "Si"=w348:bool, "No"=w347:bool, "Dis. No?"=w302:i16)
            n205 = Unbundle By Name(w308) -> ("Disable?"=w354:i16, "Si"=w345:bool, "No"=w346:bool, "Dis. No?"=w303:i16)
            n206 = Unbundle By Name(w309) -> ("Disable?"=w355:i16, "Si"=w341:bool, "No"=w342:bool, "Dis. No?"=w304:i16)
            n207 = Unbundle By Name(w310) -> ("Disable?"=w356:i16, "Si"=w344:bool, "No"=w343:bool, "Dis. No?"=w305:i16)
            n208 = Unbundle By Name(w311) -> ("Disable?"=w357:i16, "Si"=w349:bool, "No"=w350:bool, "Dis. No?"=w306:i16)
            n209 = Bundle By Name(cluster=w359, "Si"=w330, "No"=w331) -> (w332:cluster{"Si":bool, "No":bool})
            n210 = Bundle By Name(cluster=w359, "Si"=w334, "No"=w333) -> (w336:cluster{"Si":bool, "No":bool})
            n211 = Bundle By Name(cluster=w359, "Si"=w340, "No"=w339) -> (w365:cluster{"Si":bool, "No":bool})
            n212 = Bundle By Name(cluster=w359, "Si"=w337, "No"=w338) -> (w364:cluster{"Si":bool, "No":bool})
            n213 = Bundle By Name(cluster=w359, "Si"=w348, "No"=w347) -> (w363:cluster{"Si":bool, "No":bool})
            n214 = Bundle By Name(cluster=w359, "Si"=w345, "No"=w346) -> (w362:cluster{"Si":bool, "No":bool})
            n215 = Bundle By Name(cluster=w359, "Si"=w341, "No"=w342) -> (w361:cluster{"Si":bool, "No":bool})
            n216 = Bundle By Name(cluster=w359, "Si"=w344, "No"=w343) -> (w360:cluster{"Si":bool, "No":bool})
            n217 = Bundle By Name(cluster=w359, "Si"=w349, "No"=w350) -> (w358:cluster{"Si":bool, "No":bool})
            n218 = local write "Si/No 1"(w332) -> ()
            n219 = local write "Si/No 2"(w336) -> ()
            n220 = local write "Si/No 3"(w365) -> ()
            n221 = local write "Si/No 4"(w364) -> ()
            n222 = local write "Si/No 5"(w363) -> ()
            n223 = local write "Si/No 6"(w362) -> ()
            n224 = local write "Si/No 7"(w361) -> ()
            n225 = local write "Si/No 8"(w360) -> ()
            n226 = local write "Si/No 9"(w358) -> ()
            n227 = property on="Si/No 2" class="Clust (strict)"("Disabled"=w335) -> ()  [unwired: 2 in, 2 out]
            n228 = property on="Si/No 3" class="Clust (strict)"("Disabled"=w351) -> ()  [unwired: 2 in, 2 out]
            n229 = property on="Si/No 4" class="Clust (strict)"("Disabled"=w352) -> ()  [unwired: 2 in, 2 out]
            n230 = property on="Si/No 5" class="Clust (strict)"("Disabled"=w353) -> ()  [unwired: 2 in, 2 out]
            n231 = property on="Si/No 6" class="Clust (strict)"("Disabled"=w354) -> ()  [unwired: 2 in, 2 out]
            n232 = property on="Si/No 7" class="Clust (strict)"("Disabled"=w355) -> ()  [unwired: 2 in, 2 out]
            n233 = property on="Si/No 8" class="Clust (strict)"("Disabled"=w356) -> ()  [unwired: 2 in, 2 out]
            n234 = property on="Si/No 9" class="Clust (strict)"("Disabled"=w357) -> ()  [unwired: 2 in, 2 out]
            n235 = property on="Si/No 1" class="Clust (strict)"("Disabled"=w329) -> ()  [unwired: 2 in, 2 out]
            n236 = property on="No" class="Bool (strict)"("Disabled"=w307) -> ()  [unwired: 2 in, 2 out]
            n237 = property on="No" class="Bool (strict)"("Disabled"=w299) -> ()  [unwired: 2 in, 2 out]
            n238 = property on="No" class="Bool (strict)"("Disabled"=w300) -> ()  [unwired: 2 in, 2 out]
            n239 = property on="No" class="Bool (strict)"("Disabled"=w301) -> ()  [unwired: 2 in, 2 out]
            n240 = property on="No" class="Bool (strict)"("Disabled"=w302) -> ()  [unwired: 2 in, 2 out]
            n241 = property on="No" class="Bool (strict)"("Disabled"=w303) -> ()  [unwired: 2 in, 2 out]
            n242 = property on="No" class="Bool (strict)"("Disabled"=w304) -> ()  [unwired: 2 in, 2 out]
            n243 = property on="No" class="Bool (strict)"("Disabled"=w305) -> ()  [unwired: 2 in, 2 out]
            n244 = property on="No" class="Bool (strict)"("Disabled"=w306) -> ()  [unwired: 2 in, 2 out]
            n245 = local read "t. 1"() -> (w295:i32)
            n246 = property on="No" class="Bool (strict)"("Visible"=FALSE) -> ()  [unwired: 2 in, 2 out]
            n247 = Tick Count (ms)() -> (millisecond timer value=w296:u32)
            "t. 2" <- w296
            n248 = Build Array (concatenate)(w298, w297) -> (w286:string[])
            n249 = case shown="True" w287 {
              tunnel: w286 -> [_ w366]
              frame False {
              }
              frame True {
                n250 = global write "Globali.vi" "Dati_report"(w366) -> ()
              }
            }
            n251 = Select(t=u16 101, s=w287, f=w290) -> (s? t:f=w289:u16)
          }
          frame 3 {
            w440 = cluster{"Si":bool, "No":bool} {"Si"=FALSE, "No"=FALSE} ("Si/No 1")
            # "RODAGGIO"
            n252 = call "Dividi tabella descrizione operazione.vi"("Numero operazione"=w375) -> ("operazioni"=w408:string[])  [unwired: 10 in]
            n253 = global read "Globali.vi" "Fase_collaudo"() -> (w371:u16)
            n254 = local read "Si/No 1"() -> (w407:cluster{"Si":bool, "No":bool})
            n255 = local read "Si/No 2"() -> (w406:cluster{"Si":bool, "No":bool})
            n256 = local read "Si/No 3"() -> (w405:cluster{"Si":bool, "No":bool})
            n257 = local read "Si/No 4"() -> (w404:cluster{"Si":bool, "No":bool})
            n258 = local read "Si/No 5"() -> (w403:cluster{"Si":bool, "No":bool})
            n259 = local read "Si/No 6"() -> (w399:cluster{"Si":bool, "No":bool})
            n260 = local read "Si/No 7"() -> (w400:cluster{"Si":bool, "No":bool})
            n261 = local read "Si/No 8"() -> (w401:cluster{"Si":bool, "No":bool})
            n262 = local read "Si/No 9"() -> (w402:cluster{"Si":bool, "No":bool})
            n263 = call "OP3_RODAGGIO.vi"("Esito 2 in"=w406, "Esito 3 in"=w405, "Esito 4 in"=w404, "Esito 5 in"=w403, "Esito 6 in"=w399, "Esito 7 in"=w400, "Esito 8 in"=w401, "Esito 9 in"=w402, "Esito 1 in"=w407, "Tasto premuto"=w374, "Tipo specifica"=w398, "Stato in"=w375, "Stato out"=w371) -> ("Dato"=w378:string[], "ANNULLA PROVA"=w367:bool, "Esito 1 out"=w397:T2, "i out"=w373:i32, "Esito 2 out"=w396:T2, "Esito 3 out"=w395:T2, "Esito 4 out"=w394:T2, "Esito 5 out"=w393:T2, "Esito 6 out"=w389:T2, "Esito 7 out"=w390:T2, "Esito 8 out"=w391:T2, "Esito 9 out"=w392:T2)  [unwired: 3 in]
            n264 = Unbundle By Name(w397) -> ("Disable?"=w410:i16, "Si"=w411:bool, "No"=w412:bool, "Dis. No?"=w388:i16)
            n265 = Unbundle By Name(w396) -> ("Disable?"=w416:i16, "Si"=w415:bool, "No"=w414:bool, "Dis. No?"=w380:i16)
            n266 = Unbundle By Name(w395) -> ("Disable?"=w432:i16, "Si"=w421:bool, "No"=w420:bool, "Dis. No?"=w381:i16)
            n267 = Unbundle By Name(w394) -> ("Disable?"=w433:i16, "Si"=w418:bool, "No"=w419:bool, "Dis. No?"=w382:i16)
            n268 = Unbundle By Name(w393) -> ("Disable?"=w434:i16, "Si"=w429:bool, "No"=w428:bool, "Dis. No?"=w383:i16)
            n269 = Unbundle By Name(w389) -> ("Disable?"=w435:i16, "Si"=w426:bool, "No"=w427:bool, "Dis. No?"=w384:i16)
            n270 = Unbundle By Name(w390) -> ("Disable?"=w436:i16, "Si"=w422:bool, "No"=w423:bool, "Dis. No?"=w385:i16)
            n271 = Unbundle By Name(w391) -> ("Disable?"=w437:i16, "Si"=w425:bool, "No"=w424:bool, "Dis. No?"=w386:i16)
            n272 = Unbundle By Name(w392) -> ("Disable?"=w438:i16, "Si"=w430:bool, "No"=w431:bool, "Dis. No?"=w387:i16)
            n273 = Bundle By Name(cluster=w440, "Si"=w411, "No"=w412) -> (w413:cluster{"Si":bool, "No":bool})
            n274 = Bundle By Name(cluster=w440, "Si"=w415, "No"=w414) -> (w417:cluster{"Si":bool, "No":bool})
            n275 = Bundle By Name(cluster=w440, "Si"=w421, "No"=w420) -> (w446:cluster{"Si":bool, "No":bool})
            n276 = Bundle By Name(cluster=w440, "Si"=w418, "No"=w419) -> (w445:cluster{"Si":bool, "No":bool})
            n277 = Bundle By Name(cluster=w440, "Si"=w429, "No"=w428) -> (w444:cluster{"Si":bool, "No":bool})
            n278 = Bundle By Name(cluster=w440, "Si"=w426, "No"=w427) -> (w443:cluster{"Si":bool, "No":bool})
            n279 = Bundle By Name(cluster=w440, "Si"=w422, "No"=w423) -> (w442:cluster{"Si":bool, "No":bool})
            n280 = Bundle By Name(cluster=w440, "Si"=w425, "No"=w424) -> (w441:cluster{"Si":bool, "No":bool})
            n281 = Bundle By Name(cluster=w440, "Si"=w430, "No"=w431) -> (w439:cluster{"Si":bool, "No":bool})
            n282 = local write "Si/No 1"(w413) -> ()
            n283 = local write "Si/No 2"(w417) -> ()
            n284 = local write "Si/No 3"(w446) -> ()
            n285 = local write "Si/No 4"(w445) -> ()
            n286 = local write "Si/No 5"(w444) -> ()
            n287 = local write "Si/No 6"(w443) -> ()
            n288 = local write "Si/No 7"(w442) -> ()
            n289 = local write "Si/No 8"(w441) -> ()
            n290 = local write "Si/No 9"(w439) -> ()
            n291 = property on="Si/No 2" class="Clust (strict)"("Disabled"=w416) -> ()  [unwired: 2 in, 2 out]
            n292 = property on="Si/No 3" class="Clust (strict)"("Disabled"=w432) -> ()  [unwired: 2 in, 2 out]
            n293 = property on="Si/No 4" class="Clust (strict)"("Disabled"=w433) -> ()  [unwired: 2 in, 2 out]
            n294 = property on="Si/No 5" class="Clust (strict)"("Disabled"=w434) -> ()  [unwired: 2 in, 2 out]
            n295 = property on="Si/No 6" class="Clust (strict)"("Disabled"=w435) -> ()  [unwired: 2 in, 2 out]
            n296 = property on="Si/No 7" class="Clust (strict)"("Disabled"=w436) -> ()  [unwired: 2 in, 2 out]
            n297 = property on="Si/No 8" class="Clust (strict)"("Disabled"=w437) -> ()  [unwired: 2 in, 2 out]
            n298 = property on="Si/No 9" class="Clust (strict)"("Disabled"=w438) -> ()  [unwired: 2 in, 2 out]
            n299 = property on="Si/No 1" class="Clust (strict)"("Disabled"=w410) -> ()  [unwired: 2 in, 2 out]
            n300 = property on="No" class="Bool (strict)"("Disabled"=w388) -> ()  [unwired: 2 in, 2 out]
            n301 = property on="No" class="Bool (strict)"("Disabled"=w380) -> ()  [unwired: 2 in, 2 out]
            n302 = property on="No" class="Bool (strict)"("Disabled"=w381) -> ()  [unwired: 2 in, 2 out]
            n303 = property on="No" class="Bool (strict)"("Disabled"=w382) -> ()  [unwired: 2 in, 2 out]
            n304 = property on="No" class="Bool (strict)"("Disabled"=w383) -> ()  [unwired: 2 in, 2 out]
            n305 = property on="No" class="Bool (strict)"("Disabled"=w384) -> ()  [unwired: 2 in, 2 out]
            n306 = property on="No" class="Bool (strict)"("Disabled"=w385) -> ()  [unwired: 2 in, 2 out]
            n307 = property on="No" class="Bool (strict)"("Disabled"=w386) -> ()  [unwired: 2 in, 2 out]
            n308 = property on="No" class="Bool (strict)"("Disabled"=w387) -> ()  [unwired: 2 in, 2 out]
            n309 = local read "t. 2"() -> (w376:i32)
            n310 = property on="No" class="Bool (strict)"("Visible"=FALSE) -> ()  [unwired: 2 in, 2 out]
            n311 = Tick Count (ms)() -> (millisecond timer value=w377:u32)
            "t. 3" <- w377
            n312 = Build Array (concatenate)(w379, w378) -> (w368:string[])
            n313 = case shown="True" w367 {
              tunnel: w368 -> [_ w447]
              frame False {
              }
              frame True {
                n314 = global write "Globali.vi" "Dati_report"(w447) -> ()
              }
            }
            n315 = Select(t=u16 101, s=w367, f=w371) -> (s? t:f=w370:u16)
          }
          frame 4 {
            w512 = cluster{"Si":bool, "No":bool} {"Si"=FALSE, "No"=FALSE} ("Si/No 1")
            # "FUNZIONAMENTO"
            n316 = call "Dividi tabella descrizione operazione.vi"("Numero operazione"=w456) -> ("operazioni"=w480:string[])  [unwired: 10 in]
            n317 = global read "Globali.vi" "Fase_collaudo"() -> (w452:u16)
            n318 = local read "Si/No 1"() -> (w479:cluster{"Si":bool, "No":bool})
            n319 = local read "Si/No 2"() -> (w478:cluster{"Si":bool, "No":bool})
            n320 = local read "Si/No 3"() -> (w477:cluster{"Si":bool, "No":bool})
            n321 = local read "Si/No 4"() -> (w476:cluster{"Si":bool, "No":bool})
            n322 = local read "Si/No 5"() -> (w475:cluster{"Si":bool, "No":bool})
            n323 = local read "Si/No 6"() -> (w471:cluster{"Si":bool, "No":bool})
            n324 = local read "Si/No 7"() -> (w472:cluster{"Si":bool, "No":bool})
            n325 = local read "Si/No 8"() -> (w473:cluster{"Si":bool, "No":bool})
            n326 = local read "Si/No 9"() -> (w474:cluster{"Si":bool, "No":bool})
            n327 = call "OP4_FUNZIONAMENTO.vi"("Esito 2 in"=w478, "Esito 3 in"=w477, "Esito 4 in"=w476, "Esito 5 in"=w475, "Esito 6 in"=w471, "Esito 7 in"=w472, "Esito 8 in"=w473, "Esito 9 in"=w474, "Esito 1 in"=w479, "Tasto premuto"=w454, "Tipo specifica"=w470, "Stato in"=w456, "Stato out"=w452) -> ("Dato"=w459:string[], "ANNULLA PROVA"=w448:bool, "Esito 1 out"=w469:T2, "i out"=w455:i32, "Esito 2 out"=w468:T2, "Esito 3 out"=w467:T2, "Esito 4 out"=w466:T2, "Esito 5 out"=w465:T2, "Esito 6 out"=w461:T2, "Esito 7 out"=w462:T2, "Esito 8 out"=w463:T2, "Esito 9 out"=w464:T2)  [unwired: 3 in]
            n328 = Unbundle By Name(w469) -> ("Disable?"=w482:i16, "Si"=w483:bool, "No"=w484:bool)
            n329 = Unbundle By Name(w468) -> ("Disable?"=w488:i16, "Si"=w487:bool, "No"=w486:bool)
            n330 = Unbundle By Name(w467) -> ("Disable?"=w504:i16, "Si"=w493:bool, "No"=w492:bool)
            n331 = Unbundle By Name(w466) -> ("Disable?"=w505:i16, "Si"=w490:bool, "No"=w491:bool)
            n332 = Unbundle By Name(w465) -> ("Disable?"=w506:i16, "Si"=w501:bool, "No"=w500:bool)
            n333 = Unbundle By Name(w461) -> ("Disable?"=w507:i16, "Si"=w498:bool, "No"=w499:bool)
            n334 = Unbundle By Name(w462) -> ("Disable?"=w508:i16, "Si"=w494:bool, "No"=w495:bool)
            n335 = Unbundle By Name(w463) -> ("Disable?"=w509:i16, "Si"=w497:bool, "No"=w496:bool)
            n336 = Unbundle By Name(w464) -> ("Disable?"=w510:i16, "Si"=w502:bool, "No"=w503:bool)
            n337 = Bundle By Name(cluster=w512, "Si"=w483, "No"=w484) -> (w485:cluster{"Si":bool, "No":bool})
            n338 = Bundle By Name(cluster=w512, "Si"=w487, "No"=w486) -> (w489:cluster{"Si":bool, "No":bool})
            n339 = Bundle By Name(cluster=w512, "Si"=w493, "No"=w492) -> (w518:cluster{"Si":bool, "No":bool})
            n340 = Bundle By Name(cluster=w512, "Si"=w490, "No"=w491) -> (w517:cluster{"Si":bool, "No":bool})
            n341 = Bundle By Name(cluster=w512, "Si"=w501, "No"=w500) -> (w516:cluster{"Si":bool, "No":bool})
            n342 = Bundle By Name(cluster=w512, "Si"=w498, "No"=w499) -> (w515:cluster{"Si":bool, "No":bool})
            n343 = Bundle By Name(cluster=w512, "Si"=w494, "No"=w495) -> (w514:cluster{"Si":bool, "No":bool})
            n344 = Bundle By Name(cluster=w512, "Si"=w497, "No"=w496) -> (w513:cluster{"Si":bool, "No":bool})
            n345 = Bundle By Name(cluster=w512, "Si"=w502, "No"=w503) -> (w511:cluster{"Si":bool, "No":bool})
            n346 = local write "Si/No 1"(w485) -> ()
            n347 = local write "Si/No 2"(w489) -> ()
            n348 = local write "Si/No 3"(w518) -> ()
            n349 = local write "Si/No 4"(w517) -> ()
            n350 = local write "Si/No 5"(w516) -> ()
            n351 = local write "Si/No 6"(w515) -> ()
            n352 = local write "Si/No 7"(w514) -> ()
            n353 = local write "Si/No 8"(w513) -> ()
            n354 = local write "Si/No 9"(w511) -> ()
            n355 = property on="Si/No 1" class="Clust (strict)"("Disabled"=w482) -> ()  [unwired: 2 in, 2 out]
            n356 = property on="Si/No 2" class="Clust (strict)"("Disabled"=w488) -> ()  [unwired: 2 in, 2 out]
            n357 = property on="Si/No 3" class="Clust (strict)"("Disabled"=w504) -> ()  [unwired: 2 in, 2 out]
            n358 = property on="Si/No 4" class="Clust (strict)"("Disabled"=w505) -> ()  [unwired: 2 in, 2 out]
            n359 = property on="Si/No 5" class="Clust (strict)"("Disabled"=w506) -> ()  [unwired: 2 in, 2 out]
            n360 = property on="Si/No 6" class="Clust (strict)"("Disabled"=w507) -> ()  [unwired: 2 in, 2 out]
            n361 = property on="Si/No 7" class="Clust (strict)"("Disabled"=w508) -> ()  [unwired: 2 in, 2 out]
            n362 = property on="Si/No 8" class="Clust (strict)"("Disabled"=w509) -> ()  [unwired: 2 in, 2 out]
            n363 = property on="Si/No 9" class="Clust (strict)"("Disabled"=w510) -> ()  [unwired: 2 in, 2 out]
            n364 = local read "t. 3"() -> (w457:i32)
            n365 = property on="No" class="Bool (strict)"("Visible"=FALSE) -> ()  [unwired: 2 in, 2 out]
            n366 = Tick Count (ms)() -> (millisecond timer value=w458:u32)
            "t. 4" <- w458
            n367 = Build Array (concatenate)(w460, w459) -> (w449:string[])
            n368 = case shown="True" w448 {
              tunnel: w449 -> [_ w519]
              frame False {
              }
              frame True {
                n369 = global write "Globali.vi" "Dati_report"(w519) -> ()
              }
            }
            n370 = Select(t=u16 101, s=w448, f=w452) -> (s? t:f=w451:u16)
          }
          frame 5 {
            w593 = cluster{"Si":bool, "No":bool} {"Si"=FALSE, "No"=FALSE} ("Si/No 1")
            # "PRESSURIZZAZIONE"
            n371 = call "Dividi tabella descrizione operazione.vi"("Numero operazione"=w528) -> ("operazioni"=w561:string[])  [unwired: 10 in]
            n372 = global read "Globali.vi" "Fase_collaudo"() -> (w524:u16)
            n373 = local read "Si/No 1"() -> (w560:cluster{"Si":bool, "No":bool})
            n374 = local read "Si/No 2"() -> (w559:cluster{"Si":bool, "No":bool})
            n375 = local read "Si/No 3"() -> (w558:cluster{"Si":bool, "No":bool})
            n376 = local read "Si/No 4"() -> (w557:cluster{"Si":bool, "No":bool})
            n377 = local read "Si/No 5"() -> (w556:cluster{"Si":bool, "No":bool})
            n378 = local read "Si/No 6"() -> (w552:cluster{"Si":bool, "No":bool})
            n379 = local read "Si/No 7"() -> (w553:cluster{"Si":bool, "No":bool})
            n380 = local read "Si/No 8"() -> (w554:cluster{"Si":bool, "No":bool})
            n381 = local read "Si/No 9"() -> (w555:cluster{"Si":bool, "No":bool})
            n382 = call "OP5_PRESSURIZZAZIONE.vi"("Esito 2 in"=w559, "Esito 3 in"=w558, "Esito 4 in"=w557, "Esito 5 in"=w556, "Esito 6 in"=w552, "Esito 7 in"=w553, "Esito 8 in"=w554, "Esito 9 in"=w555, "Esito 1 in"=w560, "Tasto premuto"=w526, "Tipo specifica"=w551, "Stato in"=w528, "Stato out"=w524) -> ("Dato"=w531:string[], "ANNULLA PROVA"=w520:bool, "Esito 1 out"=w550:T2, "i out"=w527:i32, "Esito 2 out"=w549:T2, "Esito 3 out"=w548:T2, "Esito 4 out"=w547:T2, "Esito 5 out"=w546:T2, "Esito 6 out"=w542:T2, "Esito 7 out"=w543:T2, "Esito 8 out"=w544:T2, "Esito 9 out"=w545:T2)  [unwired: 3 in]
            n383 = Unbundle By Name(w550) -> ("Disable?"=w563:i16, "Si"=w564:bool, "No"=w565:bool, "Dis. No?"=w541:i16)
            n384 = Unbundle By Name(w549) -> ("Disable?"=w569:i16, "Si"=w568:bool, "No"=w567:bool, "Dis. No?"=w533:i16)
            n385 = Unbundle By Name(w548) -> ("Disable?"=w585:i16, "Si"=w574:bool, "No"=w573:bool, "Dis. No?"=w534:i16)
            n386 = Unbundle By Name(w547) -> ("Disable?"=w586:i16, "Si"=w571:bool, "No"=w572:bool, "Dis. No?"=w535:i16)
            n387 = Unbundle By Name(w546) -> ("Disable?"=w587:i16, "Si"=w582:bool, "No"=w581:bool, "Dis. No?"=w536:i16)
            n388 = Unbundle By Name(w542) -> ("Disable?"=w588:i16, "Si"=w579:bool, "No"=w580:bool, "Dis. No?"=w537:i16)
            n389 = Unbundle By Name(w543) -> ("Disable?"=w589:i16, "Si"=w575:bool, "No"=w576:bool, "Dis. No?"=w538:i16)
            n390 = Unbundle By Name(w544) -> ("Disable?"=w590:i16, "Si"=w578:bool, "No"=w577:bool, "Dis. No?"=w539:i16)
            n391 = Unbundle By Name(w545) -> ("Disable?"=w591:i16, "Si"=w583:bool, "No"=w584:bool, "Dis. No?"=w540:i16)
            n392 = Bundle By Name(cluster=w593, "Si"=w564, "No"=w565) -> (w566:cluster{"Si":bool, "No":bool})
            n393 = Bundle By Name(cluster=w593, "Si"=w568, "No"=w567) -> (w570:cluster{"Si":bool, "No":bool})
            n394 = Bundle By Name(cluster=w593, "Si"=w574, "No"=w573) -> (w599:cluster{"Si":bool, "No":bool})
            n395 = Bundle By Name(cluster=w593, "Si"=w571, "No"=w572) -> (w598:cluster{"Si":bool, "No":bool})
            n396 = Bundle By Name(cluster=w593, "Si"=w582, "No"=w581) -> (w597:cluster{"Si":bool, "No":bool})
            n397 = Bundle By Name(cluster=w593, "Si"=w579, "No"=w580) -> (w596:cluster{"Si":bool, "No":bool})
            n398 = Bundle By Name(cluster=w593, "Si"=w575, "No"=w576) -> (w595:cluster{"Si":bool, "No":bool})
            n399 = Bundle By Name(cluster=w593, "Si"=w578, "No"=w577) -> (w594:cluster{"Si":bool, "No":bool})
            n400 = Bundle By Name(cluster=w593, "Si"=w583, "No"=w584) -> (w592:cluster{"Si":bool, "No":bool})
            n401 = local write "Si/No 1"(w566) -> ()
            n402 = local write "Si/No 2"(w570) -> ()
            n403 = local write "Si/No 3"(w599) -> ()
            n404 = local write "Si/No 4"(w598) -> ()
            n405 = local write "Si/No 5"(w597) -> ()
            n406 = local write "Si/No 6"(w596) -> ()
            n407 = local write "Si/No 7"(w595) -> ()
            n408 = local write "Si/No 8"(w594) -> ()
            n409 = local write "Si/No 9"(w592) -> ()
            n410 = property on="Si/No 2" class="Clust (strict)"("Disabled"=w569) -> ()  [unwired: 2 in, 2 out]
            n411 = property on="Si/No 3" class="Clust (strict)"("Disabled"=w585) -> ()  [unwired: 2 in, 2 out]
            n412 = property on="Si/No 4" class="Clust (strict)"("Disabled"=w586) -> ()  [unwired: 2 in, 2 out]
            n413 = property on="Si/No 5" class="Clust (strict)"("Disabled"=w587) -> ()  [unwired: 2 in, 2 out]
            n414 = property on="Si/No 6" class="Clust (strict)"("Disabled"=w588) -> ()  [unwired: 2 in, 2 out]
            n415 = property on="Si/No 7" class="Clust (strict)"("Disabled"=w589) -> ()  [unwired: 2 in, 2 out]
            n416 = property on="Si/No 8" class="Clust (strict)"("Disabled"=w590) -> ()  [unwired: 2 in, 2 out]
            n417 = property on="Si/No 9" class="Clust (strict)"("Disabled"=w591) -> ()  [unwired: 2 in, 2 out]
            n418 = property on="Si/No 1" class="Clust (strict)"("Disabled"=w563) -> ()  [unwired: 2 in, 2 out]
            n419 = property on="No" class="Bool (strict)"("Disabled"=w541) -> ()  [unwired: 2 in, 2 out]
            n420 = property on="No" class="Bool (strict)"("Disabled"=w533) -> ()  [unwired: 2 in, 2 out]
            n421 = property on="No" class="Bool (strict)"("Disabled"=w534) -> ()  [unwired: 2 in, 2 out]
            n422 = property on="No" class="Bool (strict)"("Disabled"=w535) -> ()  [unwired: 2 in, 2 out]
            n423 = property on="No" class="Bool (strict)"("Disabled"=w536) -> ()  [unwired: 2 in, 2 out]
            n424 = property on="No" class="Bool (strict)"("Disabled"=w537) -> ()  [unwired: 2 in, 2 out]
            n425 = property on="No" class="Bool (strict)"("Disabled"=w538) -> ()  [unwired: 2 in, 2 out]
            n426 = property on="No" class="Bool (strict)"("Disabled"=w539) -> ()  [unwired: 2 in, 2 out]
            n427 = property on="No" class="Bool (strict)"("Disabled"=w540) -> ()  [unwired: 2 in, 2 out]
            n428 = local read "t. 4"() -> (w529:i32)
            n429 = property on="No" class="Bool (strict)"("Visible"=TRUE) -> ()  [unwired: 2 in, 2 out]
            n430 = Tick Count (ms)() -> (millisecond timer value=w530:u32)
            "t. 5" <- w530
            n431 = Build Array (concatenate)(w532, w531) -> (w521:string[])
            n432 = case shown="True" w520 {
              tunnel: w521 -> [_ w600]
              frame False {
              }
              frame True {
                n433 = global write "Globali.vi" "Dati_report"(w600) -> ()
              }
            }
            n434 = Select(t=u16 101, s=w520, f=w524) -> (s? t:f=w523:u16)
          }
          frame 6 {
            w677 = cluster{"Si":bool, "No":bool} {"Si"=FALSE, "No"=FALSE} ("Si/No 1")
            # "Rimango in fase 6 fino a quando non vengono\nflaggati tutti gli esiti di scarico, allora passo alla\nfase 100 (salva report buoni)"
            # "SCARICO"
            n435 = call "Dividi tabella descrizione operazione.vi"("Numero operazione"=w610) -> ("operazioni"=w645:string[])  [unwired: 10 in]
            n436 = global read "Globali.vi" "Fase_collaudo"() -> (w613:u16)
            n437 = local read "Si/No 1"() -> (w644:cluster{"Si":bool, "No":bool})
            n438 = local read "Si/No 2"() -> (w643:cluster{"Si":bool, "No":bool})
            n439 = local read "Si/No 3"() -> (w642:cluster{"Si":bool, "No":bool})
            n440 = local read "Si/No 4"() -> (w641:cluster{"Si":bool, "No":bool})
            n441 = local read "Si/No 5"() -> (w640:cluster{"Si":bool, "No":bool})
            n442 = local read "Si/No 6"() -> (w636:cluster{"Si":bool, "No":bool})
            n443 = local read "Si/No 7"() -> (w637:cluster{"Si":bool, "No":bool})
            n444 = local read "Si/No 8"() -> (w638:cluster{"Si":bool, "No":bool})
            n445 = local read "Si/No 9"() -> (w639:cluster{"Si":bool, "No":bool})
            n446 = call "OP6_SCARICO.vi"("Esito 2 in"=w643, "Esito 3 in"=w642, "Esito 4 in"=w641, "Esito 5 in"=w640, "Esito 6 in"=w636, "Esito 7 in"=w637, "Esito 8 in"=w638, "Esito 9 in"=w639, "Esito 1 in"=w644, "Tasto premuto"=w608, "Tipo specifica"=w635, "Stato in"=w610, "Stato out"=w613) -> ("scrivi"=w606:bool, "Dato"=w615:string[], "Esito 1 out"=w634:T2, "i out"=w609:i32, "Esito 2 out"=w633:T2, "Esito 3 out"=w632:T2, "Esito 4 out"=w631:T2, "Esito 5 out"=w630:T2, "Esito 6 out"=w626:T2, "Esito 7 out"=w627:T2, "Esito 8 out"=w628:T2, "Esito 9 out"=w629:T2)  [unwired: 2 in, 1 out]
            n447 = Unbundle By Name(w634) -> ("Disable?"=w647:i16, "Si"=w648:bool, "No"=w649:bool, "Dis. No?"=w625:i16)
            n448 = Unbundle By Name(w633) -> ("Disable?"=w653:i16, "Si"=w652:bool, "No"=w651:bool, "Dis. No?"=w617:i16)
            n449 = Unbundle By Name(w632) -> ("Disable?"=w669:i16, "Si"=w658:bool, "No"=w657:bool, "Dis. No?"=w618:i16)
            n450 = Unbundle By Name(w631) -> ("Disable?"=w670:i16, "Si"=w655:bool, "No"=w656:bool, "Dis. No?"=w619:i16)
            n451 = Unbundle By Name(w630) -> ("Disable?"=w671:i16, "Si"=w666:bool, "No"=w665:bool, "Dis. No?"=w620:i16)
            n452 = Unbundle By Name(w626) -> ("Disable?"=w672:i16, "Si"=w663:bool, "No"=w664:bool, "Dis. No?"=w621:i16)
            n453 = Unbundle By Name(w627) -> ("Disable?"=w673:i16, "Si"=w659:bool, "No"=w660:bool, "Dis. No?"=w622:i16)
            n454 = Unbundle By Name(w628) -> ("Disable?"=w674:i16, "Si"=w662:bool, "No"=w661:bool, "Dis. No?"=w623:i16)
            n455 = Unbundle By Name(w629) -> ("Disable?"=w675:i16, "Si"=w667:bool, "No"=w668:bool, "Dis. No?"=w624:i16)
            n456 = Bundle By Name(cluster=w677, "Si"=w648, "No"=w649) -> (w650:cluster{"Si":bool, "No":bool})
            n457 = Bundle By Name(cluster=w677, "Si"=w652, "No"=w651) -> (w654:cluster{"Si":bool, "No":bool})
            n458 = Bundle By Name(cluster=w677, "Si"=w658, "No"=w657) -> (w683:cluster{"Si":bool, "No":bool})
            n459 = Bundle By Name(cluster=w677, "Si"=w655, "No"=w656) -> (w682:cluster{"Si":bool, "No":bool})
            n460 = Bundle By Name(cluster=w677, "Si"=w666, "No"=w665) -> (w681:cluster{"Si":bool, "No":bool})
            n461 = Bundle By Name(cluster=w677, "Si"=w663, "No"=w664) -> (w680:cluster{"Si":bool, "No":bool})
            n462 = Bundle By Name(cluster=w677, "Si"=w659, "No"=w660) -> (w679:cluster{"Si":bool, "No":bool})
            n463 = Bundle By Name(cluster=w677, "Si"=w662, "No"=w661) -> (w678:cluster{"Si":bool, "No":bool})
            n464 = Bundle By Name(cluster=w677, "Si"=w667, "No"=w668) -> (w676:cluster{"Si":bool, "No":bool})
            n465 = local write "Si/No 1"(w650) -> ()
            n466 = local write "Si/No 2"(w654) -> ()
            n467 = local write "Si/No 3"(w683) -> ()
            n468 = local write "Si/No 4"(w682) -> ()
            n469 = local write "Si/No 5"(w681) -> ()
            n470 = local write "Si/No 6"(w680) -> ()
            n471 = local write "Si/No 7"(w679) -> ()
            n472 = local write "Si/No 8"(w678) -> ()
            n473 = local write "Si/No 9"(w676) -> ()
            n474 = property on="Si/No 2" class="Clust (strict)"("Disabled"=w653) -> ()  [unwired: 2 in, 2 out]
            n475 = property on="Si/No 3" class="Clust (strict)"("Disabled"=w669) -> ()  [unwired: 2 in, 2 out]
            n476 = property on="Si/No 4" class="Clust (strict)"("Disabled"=w670) -> ()  [unwired: 2 in, 2 out]
            n477 = property on="Si/No 5" class="Clust (strict)"("Disabled"=w671) -> ()  [unwired: 2 in, 2 out]
            n478 = property on="Si/No 6" class="Clust (strict)"("Disabled"=w672) -> ()  [unwired: 2 in, 2 out]
            n479 = property on="Si/No 7" class="Clust (strict)"("Disabled"=w673) -> ()  [unwired: 2 in, 2 out]
            n480 = property on="Si/No 8" class="Clust (strict)"("Disabled"=w674) -> ()  [unwired: 2 in, 2 out]
            n481 = property on="Si/No 9" class="Clust (strict)"("Disabled"=w675) -> ()  [unwired: 2 in, 2 out]
            n482 = property on="Si/No 1" class="Clust (strict)"("Disabled"=w647) -> ()  [unwired: 2 in, 2 out]
            n483 = property on="No" class="Bool (strict)"("Disabled"=w625) -> ()  [unwired: 2 in, 2 out]
            n484 = property on="No" class="Bool (strict)"("Disabled"=w617) -> ()  [unwired: 2 in, 2 out]
            n485 = property on="No" class="Bool (strict)"("Disabled"=w618) -> ()  [unwired: 2 in, 2 out]
            n486 = property on="No" class="Bool (strict)"("Disabled"=w619) -> ()  [unwired: 2 in, 2 out]
            n487 = property on="No" class="Bool (strict)"("Disabled"=w620) -> ()  [unwired: 2 in, 2 out]
            n488 = property on="No" class="Bool (strict)"("Disabled"=w621) -> ()  [unwired: 2 in, 2 out]
            n489 = property on="No" class="Bool (strict)"("Disabled"=w622) -> ()  [unwired: 2 in, 2 out]
            n490 = property on="No" class="Bool (strict)"("Disabled"=w623) -> ()  [unwired: 2 in, 2 out]
            n491 = property on="No" class="Bool (strict)"("Disabled"=w624) -> ()  [unwired: 2 in, 2 out]
            n492 = global write "Globali.vi" "Fase Prot35"(FALSE ("Fase Prot35")) -> ()
            n493 = global write "Globali.vi" "Fase Scarico"(TRUE ("Fase Scarico")) -> ()
            n494 = case shown="True" w606 {
              frame False {
              }
              frame True {
                n495 = property on="solo a macchina ferma e ciclo concluso" class="Bool"("Disabled"=u8 0) -> ()  [unwired: 2 in, 2 out]
              }
            }
            n496 = Select(t=u16 100, s=w606, f=u16 6) -> (s? t:f=w604:u16)
            n497 = local read "t. 5"() -> (w611:i32)
            n498 = Tick Count (ms)() -> (millisecond timer value=w612:u32)
            "t. 6" <- w612
            n499 = Build Array (concatenate)(w616, w615) -> (w605:string[])
            n500 = global write "Globali.vi" "copia dati report"(w605) -> ()
            n501 = global write "Globali.vi" "Dati_report"(w605) -> ()
            n502 = property on="No" class="Bool (strict)"("Visible"=FALSE) -> ()  [unwired: 2 in, 2 out]
          }
          frame 7 {
            w761 = cluster{"Si":bool, "No":bool} {"Si"=FALSE, "No"=FALSE} ("Si/No 1")
            # "Rimango in fase 7 fino a quando non vengono\nflaggati tutti gli esiti di scarico, allora passo alla\nfase 100 (salva report buoni)"
            # "PROT35"
            n503 = call "Dividi tabella descrizione operazione.vi"("Numero operazione"=w695) -> ("operazioni"=w729:string[])  [unwired: 10 in]
            n504 = global read "Globali.vi" "Fase_collaudo"() -> (w700:u16)
            n505 = local read "Si/No 1"() -> (w728:cluster{"Si":bool, "No":bool})
            n506 = local read "Si/No 2"() -> (w727:cluster{"Si":bool, "No":bool})
            n507 = local read "Si/No 3"() -> (w726:cluster{"Si":bool, "No":bool})
            n508 = local read "Si/No 4"() -> (w725:cluster{"Si":bool, "No":bool})
            n509 = local read "Si/No 5"() -> (w724:cluster{"Si":bool, "No":bool})
            n510 = local read "Si/No 6"() -> (w720:cluster{"Si":bool, "No":bool})
            n511 = local read "Si/No 7"() -> (w721:cluster{"Si":bool, "No":bool})
            n512 = local read "Si/No 8"() -> (w722:cluster{"Si":bool, "No":bool})
            n513 = local read "Si/No 9"() -> (w723:cluster{"Si":bool, "No":bool})
            n514 = call "OP7_PROT35.vi"("Esito 2 in"=w727, "Esito 3 in"=w726, "Esito 4 in"=w725, "Esito 5 in"=w724, "Esito 6 in"=w720, "Esito 7 in"=w721, "Esito 8 in"=w722, "Esito 9 in"=w723, "Esito 1 in"=w728, "Tasto premuto"=w693, "Tipo specifica"=w719, "Stato in"=w695, "Stato out"=w700) -> ("scrivi"=w688:bool, "Dato"=w698:string[], "Esito 1 out"=w718:T2, "i out"=w694:i32, "Esito 2 out"=w717:T2, "Esito 3 out"=w716:T2, "Esito 4 out"=w715:T2, "Esito 5 out"=w714:T2, "Esito 6 out"=w710:T2, "Esito 7 out"=w711:T2, "Esito 8 out"=w712:T2, "Esito 9 out"=w713:T2)  [unwired: 2 in, 1 out]
            n515 = Unbundle By Name(w718) -> ("Disable?"=w731:i16, "Si"=w732:bool, "No"=w733:bool, "Dis. No?"=w709:i16)
            n516 = Unbundle By Name(w717) -> ("Disable?"=w737:i16, "Si"=w736:bool, "No"=w735:bool, "Dis. No?"=w701:i16)
            n517 = Unbundle By Name(w716) -> ("Disable?"=w753:i16, "Si"=w742:bool, "No"=w741:bool, "Dis. No?"=w702:i16)
            n518 = Unbundle By Name(w715) -> ("Disable?"=w754:i16, "Si"=w739:bool, "No"=w740:bool, "Dis. No?"=w703:i16)
            n519 = Unbundle By Name(w714) -> ("Disable?"=w755:i16, "Si"=w750:bool, "No"=w749:bool, "Dis. No?"=w704:i16)
            n520 = Unbundle By Name(w710) -> ("Disable?"=w756:i16, "Si"=w747:bool, "No"=w748:bool, "Dis. No?"=w705:i16)
            n521 = Unbundle By Name(w711) -> ("Disable?"=w757:i16, "Si"=w743:bool, "No"=w744:bool, "Dis. No?"=w706:i16)
            n522 = Unbundle By Name(w712) -> ("Disable?"=w758:i16, "Si"=w746:bool, "No"=w745:bool, "Dis. No?"=w707:i16)
            n523 = Unbundle By Name(w713) -> ("Disable?"=w759:i16, "Si"=w751:bool, "No"=w752:bool, "Dis. No?"=w708:i16)
            n524 = Bundle By Name(cluster=w761, "Si"=w732, "No"=w733) -> (w734:cluster{"Si":bool, "No":bool})
            n525 = Bundle By Name(cluster=w761, "Si"=w736, "No"=w735) -> (w738:cluster{"Si":bool, "No":bool})
            n526 = Bundle By Name(cluster=w761, "Si"=w742, "No"=w741) -> (w767:cluster{"Si":bool, "No":bool})
            n527 = Bundle By Name(cluster=w761, "Si"=w739, "No"=w740) -> (w766:cluster{"Si":bool, "No":bool})
            n528 = Bundle By Name(cluster=w761, "Si"=w750, "No"=w749) -> (w765:cluster{"Si":bool, "No":bool})
            n529 = Bundle By Name(cluster=w761, "Si"=w747, "No"=w748) -> (w764:cluster{"Si":bool, "No":bool})
            n530 = Bundle By Name(cluster=w761, "Si"=w743, "No"=w744) -> (w763:cluster{"Si":bool, "No":bool})
            n531 = Bundle By Name(cluster=w761, "Si"=w746, "No"=w745) -> (w762:cluster{"Si":bool, "No":bool})
            n532 = Bundle By Name(cluster=w761, "Si"=w751, "No"=w752) -> (w760:cluster{"Si":bool, "No":bool})
            n533 = local write "Si/No 1"(w734) -> ()
            n534 = local write "Si/No 2"(w738) -> ()
            n535 = local write "Si/No 3"(w767) -> ()
            n536 = local write "Si/No 4"(w766) -> ()
            n537 = local write "Si/No 5"(w765) -> ()
            n538 = local write "Si/No 6"(w764) -> ()
            n539 = local write "Si/No 7"(w763) -> ()
            n540 = local write "Si/No 8"(w762) -> ()
            n541 = local write "Si/No 9"(w760) -> ()
            n542 = property on="Si/No 2" class="Clust (strict)"("Disabled"=w737) -> ()  [unwired: 2 in, 2 out]
            n543 = property on="Si/No 3" class="Clust (strict)"("Disabled"=w753) -> ()  [unwired: 2 in, 2 out]
            n544 = property on="Si/No 4" class="Clust (strict)"("Disabled"=w754) -> ()  [unwired: 2 in, 2 out]
            n545 = property on="Si/No 5" class="Clust (strict)"("Disabled"=w755) -> ()  [unwired: 2 in, 2 out]
            n546 = property on="Si/No 6" class="Clust (strict)"("Disabled"=w756) -> ()  [unwired: 2 in, 2 out]
            n547 = property on="Si/No 7" class="Clust (strict)"("Disabled"=w757) -> ()  [unwired: 2 in, 2 out]
            n548 = property on="Si/No 8" class="Clust (strict)"("Disabled"=w758) -> ()  [unwired: 2 in, 2 out]
            n549 = property on="Si/No 9" class="Clust (strict)"("Disabled"=w759) -> ()  [unwired: 2 in, 2 out]
            n550 = property on="Si/No 1" class="Clust (strict)"("Disabled"=w731) -> ()  [unwired: 2 in, 2 out]
            n551 = property on="No" class="Bool (strict)"("Disabled"=w709) -> ()  [unwired: 2 in, 2 out]
            n552 = property on="No" class="Bool (strict)"("Disabled"=w701) -> ()  [unwired: 2 in, 2 out]
            n553 = property on="No" class="Bool (strict)"("Disabled"=w702) -> ()  [unwired: 2 in, 2 out]
            n554 = property on="No" class="Bool (strict)"("Disabled"=w703) -> ()  [unwired: 2 in, 2 out]
            n555 = property on="No" class="Bool (strict)"("Disabled"=w704) -> ()  [unwired: 2 in, 2 out]
            n556 = property on="No" class="Bool (strict)"("Disabled"=w705) -> ()  [unwired: 2 in, 2 out]
            n557 = property on="No" class="Bool (strict)"("Disabled"=w706) -> ()  [unwired: 2 in, 2 out]
            n558 = property on="No" class="Bool (strict)"("Disabled"=w707) -> ()  [unwired: 2 in, 2 out]
            n559 = property on="No" class="Bool (strict)"("Disabled"=w708) -> ()  [unwired: 2 in, 2 out]
            n560 = global write "Globali.vi" "Fase Prot35"(TRUE ("Fase Prot35")) -> ()
            n561 = global write "Globali.vi" "Fase Scarico"(FALSE ("Fase Scarico")) -> ()
            n562 = case shown="True" w688 {
              frame False {
              }
              frame True {
                n563 = property on="solo a macchina ferma e ciclo concluso" class="Bool"("Disabled"=u8 0) -> ()  [unwired: 2 in, 2 out]
              }
            }
            n564 = Select(t=u16 100, s=w688, f=u16 7) -> (s? t:f=w687:u16)
            n565 = local read "t. 5"() -> (w696:i32)
            n566 = Tick Count (ms)() -> (millisecond timer value=w697:u32)
            "t. 7" <- w697
            n567 = Build Array (concatenate)(w699, w698) -> (w691:string[])
            n568 = global write "Globali.vi" "copia dati report"(w691) -> ()
            n569 = global write "Globali.vi" "Dati_report"(w691) -> ()
            n570 = property on="No" class="Bool (strict)"("Visible"=FALSE) -> ()  [unwired: 2 in, 2 out]
          }
          frame 100 {
            # "SALVA DATI BUONO"
            n571 = call "Leggi dati fasi collaudo.vi"("Tipo specifica"=w769) -> ("Dati"=w770:string[])  [unwired: 10 in]
            n572 = global read "Globali.vi" "MATRICOLA"() -> (w779:string)
            n573 = global read "Globali.vi" "Part number"() -> (w778:string)
            n574 = Format Date/Time String(time format string (%c)="%m/%d/%Y") -> (date/time string=w780:string)  [unwired: 2 in]
            n575 = Build Array(w780, w779, w778) -> (w781:string[])
            n576 = Build Array (concatenate)(w781, w770) -> (w772:string[])
            n577 = flat-sequence {
              tunnel: w772 -> [w787]
              tunnel: [w787] -> w773
              tunnel: [w788] -> w771
              tunnel: w773 -> [w789]
              tunnel: w771 -> [_]
              tunnel: [0] -> w774
              frame #0 {
                n578 = global write "Globali.vi" "Scarto"(FALSE ("Scarto")) -> ()
              }
              frame #1 {
                n579 = call "Fine test.vi"("Dato"=w789) -> ("error out"=w788:errorcluster)  [unwired: 7 in, 1 out]
              }
              frame #2 {
                # "Era in fine collaudo, spostato qui"
                n580 = global write "Globali.vi" "O.F.3_OK_FINE_CICLO"(TRUE ("O.F.3_OK_FINE_CICLO")) -> ()
              }
              frame #3 {
              }
            }
            n581 = local read "t. 7"() -> (w777:i32)
            n582 = Tick Count (ms)() -> (millisecond timer value=w783:u32)
          }
          frame 101 {
            # "SALVA DATI SCARTO"
            n583 = call "Leggi dati fasi collaudo.vi"("Tipo specifica"=w792) -> ("Dati"=w793:string[])  [unwired: 10 in]
            n584 = global read "Globali.vi" "MATRICOLA"() -> (w802:string)
            n585 = global read "Globali.vi" "Part number"() -> (w801:string)
            n586 = Format Date/Time String(time format string (%c)="%m/%d/%Y") -> (date/time string=w803:string)  [unwired: 2 in]
            n587 = Build Array(w803, w802, w801) -> (w804:string[])
            n588 = Build Array (concatenate)(w804, w793) -> (w795:string[])
            n589 = flat-sequence {
              tunnel: w795 -> [w810]
              tunnel: [w810] -> w796
              tunnel: [w811] -> w794
              tunnel: w796 -> [w812]
              tunnel: w794 -> [_]
              tunnel: [0] -> w797
              frame #0 {
                n590 = global write "Globali.vi" "Scarto"(TRUE ("Scarto")) -> ()
              }
              frame #1 {
                n591 = call "Fine test.vi"("Dato"=w812) -> ("error out"=w811:errorcluster)  [unwired: 7 in, 1 out]
              }
              frame #2 {
                # "Era in fine collaudo, spostato qui"
                n592 = global write "Globali.vi" "O.F.3_OK_FINE_CICLO"(TRUE ("O.F.3_OK_FINE_CICLO")) -> ()
              }
              frame #3 {
              }
            }
            n593 = local read "t. 7"() -> (w800:i32)
            n594 = Tick Count (ms)() -> (millisecond timer value=w806:u32)
          }
          frame 8 {
            w815 = 0 ("Fase_collaudo")
            n595 = call "Pagina manutenzione avvio.vi"() -> ()  [unwired: 6 in]
          }
        }
        "AVANZAMENTO COLLAUDO" <- w60
        n596 = case shown="True" "ANNULLA PROVA" {
          frame False {
          }
          frame True {
            n597 = call "Resetta_Flag_con_annulla_prova.vi"() -> ()  [unwired: 1 in]
          }
        }
        n598 = Index Array(array=w87, index=0) -> (element=w93:T3)
        n599 = case shown="True" FALSE {
          tunnel: w93 -> [_ w824]
          tunnel: u32 500 ("milliseconds to wait") -> [_ w823]
          tunnel: w88 -> [_ w822]
          frame False {
          }
          frame True {
            n600 = case shown="1" w822 {
              tunnel: w824 -> [_ w829 w833 w839 w845 w851 w857 w863 w869 w875]
              tunnel: w823 -> [_ w826 w832 w838 w844 w850 w856 w862 w868 w874]
              frame Default {
                w825 = u8 2 ("Disabled")
                n601 = property on="Si/No 1" class="Clust (strict)"("Disabled"=w825) -> ()  [unwired: 2 in, 2 out]
                n602 = property on="Si/No 2" class="Clust (strict)"("Disabled"=w825) -> ()  [unwired: 2 in, 2 out]
                n603 = property on="Si/No 3" class="Clust (strict)"("Disabled"=w825) -> ()  [unwired: 2 in, 2 out]
                n604 = property on="Si/No 4" class="Clust (strict)"("Disabled"=w825) -> ()  [unwired: 2 in, 2 out]
                n605 = property on="Si/No 5" class="Clust (strict)"("Disabled"=w825) -> ()  [unwired: 2 in, 2 out]
                n606 = property on="Si/No 6" class="Clust (strict)"("Disabled"=w825) -> ()  [unwired: 2 in, 2 out]
                n607 = property on="Si/No 7" class="Clust (strict)"("Disabled"=w825) -> ()  [unwired: 2 in, 2 out]
                n608 = property on="Si/No 8" class="Clust (strict)"("Disabled"=w825) -> ()  [unwired: 2 in, 2 out]
                n609 = property on="Si/No 9" class="Clust (strict)"("Disabled"=w825) -> ()  [unwired: 2 in, 2 out]
              }
              frame 1 {
                w827 = u8 2 ("Disabled")
                n610 = case shown="\"F12\"" w829 {
                  tunnel: w826 -> [w830 w831 _]
                  frame "F11" {
                    n611 = Wait (ms)(milliseconds to wait=w830) -> ()  [unwired: 1 out]
                  }
                  frame "F12" {
                    n612 = Wait (ms)(milliseconds to wait=w831) -> ()  [unwired: 1 out]
                  }
                  frame Default {
                  }
                }
                n613 = property on="Si/No 1" class="Clust (strict)"("Disabled"=u8 0) -> ()  [unwired: 2 in, 2 out]
                n614 = property on="Si/No 2" class="Clust (strict)"("Disabled"=w827) -> ()  [unwired: 2 in, 2 out]
                n615 = property on="Si/No 3" class="Clust (strict)"("Disabled"=w827) -> ()  [unwired: 2 in, 2 out]
                n616 = property on="Si/No 4" class="Clust (strict)"("Disabled"=w827) -> ()  [unwired: 2 in, 2 out]
                n617 = property on="Si/No 5" class="Clust (strict)"("Disabled"=w827) -> ()  [unwired: 2 in, 2 out]
                n618 = property on="Si/No 6" class="Clust (strict)"("Disabled"=w827) -> ()  [unwired: 2 in, 2 out]
                n619 = property on="Si/No 7" class="Clust (strict)"("Disabled"=w827) -> ()  [unwired: 2 in, 2 out]
                n620 = property on="Si/No 8" class="Clust (strict)"("Disabled"=w827) -> ()  [unwired: 2 in, 2 out]
                n621 = property on="Si/No 9" class="Clust (strict)"("Disabled"=w827) -> ()  [unwired: 2 in, 2 out]
              }
              frame 2 {
                w834 = u8 2 ("Disabled")
                n622 = case shown="\"F11\"" w833 {
                  tunnel: w832 -> [w836 w837 _]
                  frame "F11" {
                    n623 = Wait (ms)(milliseconds to wait=w836) -> ()  [unwired: 1 out]
                  }
                  frame "F12" {
                    n624 = Wait (ms)(milliseconds to wait=w837) -> ()  [unwired: 1 out]
                  }
                  frame Default {
                  }
                }
                n625 = property on="Si/No 2" class="Clust (strict)"("Disabled"=u8 0) -> ()  [unwired: 2 in, 2 out]
                n626 = property on="Si/No 1" class="Clust (strict)"("Disabled"=w834) -> ()  [unwired: 2 in, 2 out]
                n627 = property on="Si/No 3" class="Clust (strict)"("Disabled"=w834) -> ()  [unwired: 2 in, 2 out]
                n628 = property on="Si/No 4" class="Clust (strict)"("Disabled"=w834) -> ()  [unwired: 2 in, 2 out]
                n629 = property on="Si/No 5" class="Clust (strict)"("Disabled"=w834) -> ()  [unwired: 2 in, 2 out]
                n630 = property on="Si/No 6" class="Clust (strict)"("Disabled"=w834) -> ()  [unwired: 2 in, 2 out]
                n631 = property on="Si/No 7" class="Clust (strict)"("Disabled"=w834) -> ()  [unwired: 2 in, 2 out]
                n632 = property on="Si/No 8" class="Clust (strict)"("Disabled"=w834) -> ()  [unwired: 2 in, 2 out]
                n633 = property on="Si/No 9" class="Clust (strict)"("Disabled"=w834) -> ()  [unwired: 2 in, 2 out]
              }
              frame 3 {
                w840 = u8 2 ("Disabled")
                n634 = case shown="\"F12\"" w839 {
                  tunnel: w838 -> [w842 w843 _]
                  frame "F11" {
                    n635 = Wait (ms)(milliseconds to wait=w842) -> ()  [unwired: 1 out]
                  }
                  frame "F12" {
                    n636 = Wait (ms)(milliseconds to wait=w843) -> ()  [unwired: 1 out]
                  }
                  frame Default {
                  }
                }
                n637 = property on="Si/No 3" class="Clust (strict)"("Disabled"=u8 0) -> ()  [unwired: 2 in, 2 out]
                n638 = property on="Si/No 2" class="Clust (strict)"("Disabled"=w840) -> ()  [unwired: 2 in, 2 out]
                n639 = property on="Si/No 1" class="Clust (strict)"("Disabled"=w840) -> ()  [unwired: 2 in, 2 out]
                n640 = property on="Si/No 4" class="Clust (strict)"("Disabled"=w840) -> ()  [unwired: 2 in, 2 out]
                n641 = property on="Si/No 5" class="Clust (strict)"("Disabled"=w840) -> ()  [unwired: 2 in, 2 out]
                n642 = property on="Si/No 6" class="Clust (strict)"("Disabled"=w840) -> ()  [unwired: 2 in, 2 out]
                n643 = property on="Si/No 7" class="Clust (strict)"("Disabled"=w840) -> ()  [unwired: 2 in, 2 out]
                n644 = property on="Si/No 8" class="Clust (strict)"("Disabled"=w840) -> ()  [unwired: 2 in, 2 out]
                n645 = property on="Si/No 9" class="Clust (strict)"("Disabled"=w840) -> ()  [unwired: 2 in, 2 out]
              }
              frame 4 {
                w846 = u8 2 ("Disabled")
                n646 = case shown="\"F11\"" w845 {
                  tunnel: w844 -> [w848 w849 _]
                  frame "F11" {
                    n647 = Wait (ms)(milliseconds to wait=w848) -> ()  [unwired: 1 out]
                  }
                  frame "F12" {
                    n648 = Wait (ms)(milliseconds to wait=w849) -> ()  [unwired: 1 out]
                  }
                  frame Default {
                  }
                }
                n649 = property on="Si/No 4" class="Clust (strict)"("Disabled"=u8 0) -> ()  [unwired: 2 in, 2 out]
                n650 = property on="Si/No 2" class="Clust (strict)"("Disabled"=w846) -> ()  [unwired: 2 in, 2 out]
                n651 = property on="Si/No 3" class="Clust (strict)"("Disabled"=w846) -> ()  [unwired: 2 in, 2 out]
                n652 = property on="Si/No 1" class="Clust (strict)"("Disabled"=w846) -> ()  [unwired: 2 in, 2 out]
                n653 = property on="Si/No 5" class="Clust (strict)"("Disabled"=w846) -> ()  [unwired: 2 in, 2 out]
                n654 = property on="Si/No 6" class="Clust (strict)"("Disabled"=w846) -> ()  [unwired: 2 in, 2 out]
                n655 = property on="Si/No 7" class="Clust (strict)"("Disabled"=w846) -> ()  [unwired: 2 in, 2 out]
                n656 = property on="Si/No 8" class="Clust (strict)"("Disabled"=w846) -> ()  [unwired: 2 in, 2 out]
                n657 = property on="Si/No 9" class="Clust (strict)"("Disabled"=w846) -> ()  [unwired: 2 in, 2 out]
              }
              frame 5 {
                w852 = u8 2 ("Disabled")
                n658 = case shown="\"F11\"" w851 {
                  tunnel: w850 -> [w854 w855 _]
                  frame "F11" {
                    n659 = Wait (ms)(milliseconds to wait=w854) -> ()  [unwired: 1 out]
                  }
                  frame "F12" {
                    n660 = Wait (ms)(milliseconds to wait=w855) -> ()  [unwired: 1 out]
                  }
                  frame Default {
                  }
                }
                n661 = property on="Si/No 5" class="Clust (strict)"("Disabled"=u8 0) -> ()  [unwired: 2 in, 2 out]
                n662 = property on="Si/No 2" class="Clust (strict)"("Disabled"=w852) -> ()  [unwired: 2 in, 2 out]
                n663 = property on="Si/No 3" class="Clust (strict)"("Disabled"=w852) -> ()  [unwired: 2 in, 2 out]
                n664 = property on="Si/No 4" class="Clust (strict)"("Disabled"=w852) -> ()  [unwired: 2 in, 2 out]
                n665 = property on="Si/No 1" class="Clust (strict)"("Disabled"=w852) -> ()  [unwired: 2 in, 2 out]
                n666 = property on="Si/No 6" class="Clust (strict)"("Disabled"=w852) -> ()  [unwired: 2 in, 2 out]
                n667 = property on="Si/No 7" class="Clust (strict)"("Disabled"=w852) -> ()  [unwired: 2 in, 2 out]
                n668 = property on="Si/No 8" class="Clust (strict)"("Disabled"=w852) -> ()  [unwired: 2 in, 2 out]
                n669 = property on="Si/No 9" class="Clust (strict)"("Disabled"=w852) -> ()  [unwired: 2 in, 2 out]
              }
              frame 6 {
                w858 = u8 2 ("Disabled")
                n670 = case shown="\"F11\"" w857 {
                  tunnel: w856 -> [w860 w861 _]
                  frame "F11" {
                    n671 = Wait (ms)(milliseconds to wait=w860) -> ()  [unwired: 1 out]
                  }
                  frame "F12" {
                    n672 = Wait (ms)(milliseconds to wait=w861) -> ()  [unwired: 1 out]
                  }
                  frame Default {
                  }
                }
                n673 = property on="Si/No 6" class="Clust (strict)"("Disabled"=u8 0) -> ()  [unwired: 2 in, 2 out]
                n674 = property on="Si/No 2" class="Clust (strict)"("Disabled"=w858) -> ()  [unwired: 2 in, 2 out]
                n675 = property on="Si/No 3" class="Clust (strict)"("Disabled"=w858) -> ()  [unwired: 2 in, 2 out]
                n676 = property on="Si/No 4" class="Clust (strict)"("Disabled"=w858) -> ()  [unwired: 2 in, 2 out]
                n677 = property on="Si/No 5" class="Clust (strict)"("Disabled"=w858) -> ()  [unwired: 2 in, 2 out]
                n678 = property on="Si/No 1" class="Clust (strict)"("Disabled"=w858) -> ()  [unwired: 2 in, 2 out]
                n679 = property on="Si/No 7" class="Clust (strict)"("Disabled"=w858) -> ()  [unwired: 2 in, 2 out]
                n680 = property on="Si/No 8" class="Clust (strict)"("Disabled"=w858) -> ()  [unwired: 2 in, 2 out]
                n681 = property on="Si/No 9" class="Clust (strict)"("Disabled"=w858) -> ()  [unwired: 2 in, 2 out]
              }
              frame 7 {
                w864 = u8 2 ("Disabled")
                n682 = case shown="\"F11\"" w863 {
                  tunnel: w862 -> [w866 w867 _]
                  frame "F11" {
                    n683 = Wait (ms)(milliseconds to wait=w866) -> ()  [unwired: 1 out]
                  }
                  frame "F12" {
                    n684 = Wait (ms)(milliseconds to wait=w867) -> ()  [unwired: 1 out]
                  }
                  frame Default {
                  }
                }
                n685 = property on="Si/No 7" class="Clust (strict)"("Disabled"=u8 0) -> ()  [unwired: 2 in, 2 out]
                n686 = property on="Si/No 2" class="Clust (strict)"("Disabled"=w864) -> ()  [unwired: 2 in, 2 out]
                n687 = property on="Si/No 3" class="Clust (strict)"("Disabled"=w864) -> ()  [unwired: 2 in, 2 out]
                n688 = property on="Si/No 4" class="Clust (strict)"("Disabled"=w864) -> ()  [unwired: 2 in, 2 out]
                n689 = property on="Si/No 5" class="Clust (strict)"("Disabled"=w864) -> ()  [unwired: 2 in, 2 out]
                n690 = property on="Si/No 6" class="Clust (strict)"("Disabled"=w864) -> ()  [unwired: 2 in, 2 out]
                n691 = property on="Si/No 1" class="Clust (strict)"("Disabled"=w864) -> ()  [unwired: 2 in, 2 out]
                n692 = property on="Si/No 8" class="Clust (strict)"("Disabled"=w864) -> ()  [unwired: 2 in, 2 out]
                n693 = property on="Si/No 9" class="Clust (strict)"("Disabled"=w864) -> ()  [unwired: 2 in, 2 out]
              }
              frame 8 {
                w870 = u8 2 ("Disabled")
                n694 = case shown="\"F11\"" w869 {
                  tunnel: w868 -> [w872 w873 _]
                  frame "F11" {
                    n695 = Wait (ms)(milliseconds to wait=w872) -> ()  [unwired: 1 out]
                  }
                  frame "F12" {
                    n696 = Wait (ms)(milliseconds to wait=w873) -> ()  [unwired: 1 out]
                  }
                  frame Default {
                  }
                }
                n697 = property on="Si/No 8" class="Clust (strict)"("Disabled"=u8 0) -> ()  [unwired: 2 in, 2 out]
                n698 = property on="Si/No 2" class="Clust (strict)"("Disabled"=w870) -> ()  [unwired: 2 in, 2 out]
                n699 = property on="Si/No 3" class="Clust (strict)"("Disabled"=w870) -> ()  [unwired: 2 in, 2 out]
                n700 = property on="Si/No 4" class="Clust (strict)"("Disabled"=w870) -> ()  [unwired: 2 in, 2 out]
                n701 = property on="Si/No 5" class="Clust (strict)"("Disabled"=w870) -> ()  [unwired: 2 in, 2 out]
                n702 = property on="Si/No 6" class="Clust (strict)"("Disabled"=w870) -> ()  [unwired: 2 in, 2 out]
                n703 = property on="Si/No 7" class="Clust (strict)"("Disabled"=w870) -> ()  [unwired: 2 in, 2 out]
                n704 = property on="Si/No 1" class="Clust (strict)"("Disabled"=w870) -> ()  [unwired: 2 in, 2 out]
                n705 = property on="Si/No 9" class="Clust (strict)"("Disabled"=w870) -> ()  [unwired: 2 in, 2 out]
              }
              frame 9 {
                w876 = u8 2 ("Disabled")
                n706 = case shown="\"F11\"" w875 {
                  tunnel: w874 -> [w878 w879 _]
                  frame "F11" {
                    n707 = Wait (ms)(milliseconds to wait=w878) -> ()  [unwired: 1 out]
                  }
                  frame "F12" {
                    n708 = Wait (ms)(milliseconds to wait=w879) -> ()  [unwired: 1 out]
                  }
                  frame Default {
                  }
                }
                n709 = property on="Si/No 9" class="Clust (strict)"("Disabled"=u8 0) -> ()  [unwired: 2 in, 2 out]
                n710 = property on="Si/No 2" class="Clust (strict)"("Disabled"=w876) -> ()  [unwired: 2 in, 2 out]
                n711 = property on="Si/No 3" class="Clust (strict)"("Disabled"=w876) -> ()  [unwired: 2 in, 2 out]
                n712 = property on="Si/No 4" class="Clust (strict)"("Disabled"=w876) -> ()  [unwired: 2 in, 2 out]
                n713 = property on="Si/No 5" class="Clust (strict)"("Disabled"=w876) -> ()  [unwired: 2 in, 2 out]
                n714 = property on="Si/No 6" class="Clust (strict)"("Disabled"=w876) -> ()  [unwired: 2 in, 2 out]
                n715 = property on="Si/No 7" class="Clust (strict)"("Disabled"=w876) -> ()  [unwired: 2 in, 2 out]
                n716 = property on="Si/No 8" class="Clust (strict)"("Disabled"=w876) -> ()  [unwired: 2 in, 2 out]
                n717 = property on="Si/No 9" class="Clust (strict)"("Disabled"=w876) -> ()  [unwired: 2 in, 2 out]
              }
            }
          }
        }
        n718 = Not Equal?(x="", y=w30) -> (x != y?=w31:bool)
        n719 = property on="Testo segnalazioni" class="Str"("Blinking"=w31) -> ()  [unwired: 2 in, 2 out]
        n720 = global read "Globali.vi" "SCARICO_A"() -> (w110:bool)
        n721 = global read "Globali.vi" "SCARICO_B"() -> (w111:bool)
        n722 = Build Array("Comandi manuali", "Pagina parametri", "Pagina scarti", "Pagina diagnostica", "Login", "Pagina misure") -> (w128:bool[])
        n723 = global write "Globali.vi" "0. 0"("Comandi manuali") -> ()
        n724 = call "Cambio Pagina.vi"("pagina in"=w129, "pulsanti"=w128) -> ("pagina out"=→"pagina out":u8, "premuto"=w121:bool)
        n725 = Not(x=w110) -> (.not. x?=w106:bool)
        n726 = Not(x=w111) -> (.not. x?=w107:bool)
        n727 = Not(x=w111) -> (.not. x?=w109:bool)
        n728 = Not(x=w121) -> (.not. x?=w127:bool)
        "forza chiusura" <- w127
        n729 = And(x=w106, y=w107) -> (x .and. y?=→"PROT35":bool)
        n730 = And(x=w110, y=w109) -> (x .and. y?=→"W90":bool)
        n731 = And(x=w110, y=w111) -> (x .and. y?=→"10W30":bool)
        n732 = global read "Globali.vi" "S_PAUSA"() -> (w50:bool)
        n733 = global read "Globali.vi" "S_CARRO_IN_POSIZ_AAT"() -> (w35:bool)
        n734 = Compound Arithmetic op=OR(w127, w122) -> (w105:bool)
        n735 = global read "Globali.vi" "S_CARRO_IN_POSIZ_RP3000"() -> (w34:bool)
        n736 = case shown="\"RP3000\"" w97 {
          tunnel: [w883 w887 w891] -> w120
          frame "RP3000" {
            n737 = global read "Globali.vi" "V_TEMP_OLIO_RP3000"() -> (w883:sgl)
            n738 = property on="PRESSIONE RICIRCOLO" class="Slide (strict)"("Visible"=FALSE) -> ()  [unwired: 2 in, 2 out]
            n739 = property on="TEMPERATURA CUSCIN." class="Slide (strict)"("Visible"=FALSE) -> ()  [unwired: 2 in, 2 out]
            n740 = property on="PORTATA RICIRCOLO" class="Slide (strict)"("Visible"=FALSE) -> ()  [unwired: 2 in, 2 out]
          }
          frame "AAT_2", Default {
            n741 = global read "Globali.vi" "V_TEMP_OLIO_AAT_2"() -> (w887:sgl)
            n742 = property on="PRESSIONE RICIRCOLO" class="Slide (strict)"("Visible"=TRUE) -> ()  [unwired: 2 in, 2 out]
            n743 = property on="TEMPERATURA CUSCIN." class="Slide (strict)"("Visible"=TRUE) -> ()  [unwired: 2 in, 2 out]
            n744 = property on="PORTATA RICIRCOLO" class="Slide (strict)"("Visible"=TRUE) -> ()  [unwired: 2 in, 2 out]
          }
          frame "AAT_1_3_4" {
            n745 = global read "Globali.vi" "V_TEMP_OLIO_AAT_1_3_4"() -> (w891:sgl)
            n746 = property on="PRESSIONE RICIRCOLO" class="Slide (strict)"("Visible"=FALSE) -> ()  [unwired: 2 in, 2 out]
            n747 = property on="TEMPERATURA CUSCIN." class="Slide (strict)"("Visible"=TRUE) -> ()  [unwired: 2 in, 2 out]
            n748 = property on="PORTATA RICIRCOLO" class="Slide (strict)"("Visible"=FALSE) -> ()  [unwired: 2 in, 2 out]
          }
        }
        "TEMPERATURA OLIO COPPA" <- w120
        n749 = Not(x=w105) -> (.not. x?=w104:bool)
        n750 = local write "Prova"(w104) -> ()
        n751 = Select(t="RIPRENDI PROVA", s=w50, f="SOSPENDI PROVA") -> (s? t:f=w54:string)
        n752 = property on="SOSPENDI PROVA" class="Bool (strict)"("BoolText.Text"=w54) -> ()  [unwired: 2 in, 2 out]
        n753 = Wait Until Next ms Multiple(millisecond multiple=u32 250) -> ()  [unwired: 1 out]
        n754 = Not(x=w35) -> (.not. x?=→"CARRO IN POSIZIONE AAT":bool)
        n755 = Not(x=w34) -> (.not. x?=→"CARRO IN POSIZIONE RP3000":bool)
        n756 = global read "Globali.vi" "V_COPPIA_ASSE_TRASCINAM"() -> (→"COPPIA ASSE":sgl)
        n757 = global read "Globali.vi" "ROTAZIONE_SX"() -> (w85:bool)
        "Rotaz.SX" <- w85
        n758 = global read "Globali.vi" "VI_VEL_MOT"() -> (→"VELOCITA' MOTORE":u16)
        n759 = global read "Globali.vi" "V_TEMP_AMBIENTE"() -> (→"TEMPERATURA AMBIENTE":sgl)
        n760 = global read "Globali.vi" "V_TEMP_CUSCINETTO_AAT"() -> (→"TEMPERATURA CUSCIN.":sgl)
        n761 = global read "Globali.vi" "V_PORTATA_RICIRCOLO"() -> (→"PORTATA RICIRCOLO":sgl)
        n762 = global read "Globali.vi" "V_PRESS_OLIO_RICIRCOLO"() -> (→"PRESSIONE RICIRCOLO":sgl)
        n763 = global read "Globali.vi" "S_TRAZIONE_INSERITA"() -> (→"Trazione inserita":bool)
        n764 = global read "Globali.vi" "V_PRESSURIZZAZIONE"() -> (→"PRESSURIZZAZIONE":sgl)
        n765 = global read "Globali.vi" "V_PRESS_ARIA_6_BAR"() -> (→"PRESSIONE ARIA 6 BAR":sgl)
        n766 = global read "Globali.vi" "V_TEMP_OLIO_10W30"() -> (→"TEMPERATURA OLIO 10W30":sgl)
        n767 = global read "Globali.vi" "V_TEMP_OLIO_10W90"() -> (→"TEMPERATURA OLIO W90":sgl)
        n768 = global read "Globali.vi" "S_AUTO"() -> (w83:bool)
        "S_AUTO" <- w83
        n769 = Select(t=u32 0, s=w50, f=u32 16448250) -> (s? t:f=w53:u32)
        n770 = property on="SOSPENDI PROVA" class="Bool (strict)"("BoolText.TextColor"=w53) -> ()  [unwired: 2 in, 2 out]
        n771 = case shown="True" "stop 2" {
          frame False {
            n772 = local write "stop 2"(FALSE ("stop 2")) -> ()
          }
          frame True {
            n773 = call "PowerOff.vi"() -> ()  [unwired: 1 in]
            n774 = local write "stop 2"(FALSE ("stop 2")) -> ()
          }
        }
        n775 = global read "Globali.vi" "CICLO_IN_CORSO"() -> (w44:bool)
        n776 = global read "Globali.vi" "PLC->PC"() -> (w75:u16[])
        n777 = case shown="True" w83 {
          frame True {
            n778 = property on="Login" class="Bool"("Disabled"=u8 2) -> ()  [unwired: 2 in, 2 out]
          }
          frame False {
            n779 = property on="Login" class="Bool"("Disabled"=u8 0) -> ()  [unwired: 2 in, 2 out]
          }
        }
        n780 = Not(x=w85) -> (.not. x?=→"Rotaz.DX":bool)
        n781 = call "Dividi_testo_su_più_righe.vi"("Lungh.riga"=70, "Array"=w64) -> ("Array 2"=w63:string[])  [unwired: 9 in]
        n782 = global read "Globali.vi" "t. Step"() -> (→"t. Step":i32)
        n783 = global read "Globali.vi" "t. tot."() -> (→"t. tot.":i32)
        n784 = Subtract(x=w73, y=w61) -> (x-y=w72:u32)
        n785 = Subtract(x=w65, y=w101) -> (x-y=w66:u32)
        n786 = case shown="False" w50 {
          frame False {
            n787 = property on="SOSPENDI PROVA" class="Bool (strict)"("Colors [4]"=cluster{u32, u32}[] [{1985280, 1985280}, {1985280, 1985280}, {16777216, 16777216}, {16777216, 16777216}]) -> ()  [unwired: 2 in, 2 out]
          }
          frame True {
            n788 = property on="SOSPENDI PROVA" class="Bool (strict)"("Colors [4]"=cluster{u32, u32}[] [{16776960, 16776960}, {16776960, 16776960}, {16777216, 16777216}, {16777216, 16777216}]) -> ()  [unwired: 2 in, 2 out]
          }
        }
        n789 = Number To Decimal String(number=w75) -> (decimal integer string=→"PLC->PC":string[])  [unwired: 1 in]
        n790 = Insert Into Array(array=string[][] [["", "", "", "", ""], ["", "", "", "", ""], ["", "", "", "", ""], ["", "", "", "", ""], ["", "", "", "", ""], ["", "", "", "", ""], ["", "", "", "", ""], ["", "", "", "", ""], ["", "", "", "", ""], ["", "", "", "", ""], ["", "", "", "", ""], ["", "", "", "", ""], ["", "", "", "", ""], ["", "", "", "", ""], ["", "", "", "", ""], ["", "", "", "", ""], ["", "", "", "", ""], ["", "", "", "", ""], ["", "", "", "", ""], ["", "", "", "", ""], ["", "", "", "", ""], ["", "", "", "", ""], ["", "", "", "", ""], ["", "", "", "", ""], ["", "", "", "", ""], ["", "", "", "", ""], ["", "", "", "", ""], ["", "", "", "", ""], ["", "", "", "", ""], ["", "", "", "", ""], ["", "", "", "", ""], ["", "", "", "", ""], ["", "", "", "", ""], ["", "", "", "", ""], ["", "", "", "", ""]] ("operazioni 2"), index (col)=2 ("disabled index (col)"), new element=w63) -> (→"operazioni":string[][])  [unwired: 1 in]
        n791 = Divide(x=w72, y=u32 1000) -> ()  [unwired: 1 out]
        n792 = Divide(x=w66, y=u32 1000) -> ()  [unwired: 1 out]
        n793 = Select(t=2, s=w44, f=0) -> (s? t:f=w41:i32)
        n794 = property on="Comandi manuali" class="Bool"("Disabled"=w41) -> ()  [unwired: 2 in, 2 out]
        n795 = property on="Pagina diagnostica" class="Bool"("Disabled"=w41) -> ()  [unwired: 2 in, 2 out]
        n796 = property on="stop" class="Bool (strict)"("Disabled"=w41) -> ()  [unwired: 2 in, 2 out]
        n797 = property on="stop 2" class="Bool (strict)"("Disabled"=w41) -> ()  [unwired: 2 in, 2 out]
      }
    }
  }
  n798 = global read "Globali.vi" "Versione SW"() -> (→"Versione SW":dbl)
  n799 = call "Leggi file testi.vi"("Numero riga"=0) -> ("Testo"=→"Linea":string)  [unwired: 3 in, 1 out]
  n800 = call "Carica immagine.vi"("Immagine JPG"="Logo cliente.jpg") -> ("altezza"=w4:i16, "larghezza"=w5:i16, "Picture"=→"Picture":picture)  [unwired: 2 in]
  n801 = Bundle("larghezza"=w5, "altezza"=w4) -> (w3:cluster{"larghezza":i16, "altezza":i16})  [unwired: 1 in]
  n802 = property on="Picture" class="Pict"("Draw Area Size"=w3) -> ()  [unwired: 2 in, 2 out]
  n803 = global write "Globali.vi" "0. 1"(TRUE ("0. 1")) -> ()
  n804 = property on="solo a macchina ferma e ciclo concluso" class="Bool"("Disabled"=u8 2) -> ()  [unwired: 2 in, 2 out]
  n805 = call-poly <vilib>:"Close Input Device.vi"("error in (no error)"=w12, "device ID"=w11) -> ()  [unwired: 8 in, 1 out]
